vi "USBCam+Stage.vi"() -> ()   [LabVIEW 2014]
doc: "This is the main user interface of the Raman spectroscopy system."
uses:
  TypeDef/States.ctl
  C:/Users/light/Desktop/SI+Raman/Labview/Raman/dll/Thorlabs.MotionControl.Controls.dll
  dll/Thorlabs.MotionControl.Controls.dll
  C:/Users/light/Desktop/SI+Raman/Labview/Raman/dll/ThorLabs.MotionControl.KCube.DCServoCLI.dll
  dll/ThorLabs.MotionControl.KCube.DCServoCLI.dll
  TypeDef/StageDeviceOut.ctl
  TypeDef/StageHandleIn.ctl
  <vilib>/Utility/miscctls.llb/LVPoint32TypeDef.ctl
  TypeDef/StageSelect.ctl
  TypeDef/LaserSpot.ctl
panel:
  out "Spot Y":dbl
  out "Spot X":dbl
  in  "Box":cluster{"Width":dbl, " Height":dbl}={"Width"=200.0, " Height"=214.0}
  out "Total_Frame_Y":dbl
  out "Total_Frame_X":dbl
  out "Frame_Y":dbl
  out "Frame_X":dbl
  in  "Destination":dbl=12.0
  in  "Save Path":path=path "C:/Users/light/Desktop/Chuanzhen/test"
  in  "Scan":bool
  in  "Velocity: X and Y axis":T1(radio)=enum."0.05mm"
  in  "MoveTo":bool
  in  "Jogstep of Z axis":T2(radio)=enum."10step"
  in  "Z axis_d":bool
  in  "Z axis_u":bool
  in  "Y axis_F":bool
  in  "Y axis_B":bool
  out "Y_axis":dbl
  out "X_axis":dbl
  out "Z_axis":dbl
  in  "X axis_L":bool
  in  "X axis_R":bool
  in  "Down":bool
  in  "Top":bool
  in  "Right":bool
  in  "Left":bool
  in  "Snap":bool
  out "Boolean":bool
  in  "Pixel Size Y (um)":dbl=0.0877
  in  "LaserSpot":bool
  in  "Pixel Size X (um)":dbl=0.0877
  in  "Aim":bool
  out "Initialization finished":bool
  out "ZoomRatio":dbl format="%#_2g"
  out "Live video":picture caption="600 x 480"
  in  "Camera ID":u32
  out "Bits/Pixel":i32=8
  in  "Autogain":bool
  in  "Master Gain":i32(slide) min=0 max=100 scale=0.0..100.0
  in  "Hotpixel correction 2":bool
  in  "Blacklevel compensation":bool
  in  "Edge Filter":i32(ring)=2 items=["High"=1, "Low"=2]
  in  "Edge Filter Enable / Disable":bool
  in  "Exposure time (ms)":dbl(slide)=11.094175438596492 min=0.008982456140350877 max=101.68743859649123 step=0.05487719298245614 scale=0.008982456140350877..101.68743859649123 scale format="%#.3g"
  in  "Pixel clock":i32(slide)=20 min=7 max=86 scale=7.0..86.0
  in  "Frame rate":dbl(slide)=9.827169720568149 min=0.5 max=17.288905497022668 step=5.487719298245614e-05 scale=0.5..17.288905497022668 scale format="%^#_3g"
  in  "Blacklevel Offset":i32(slide) min=0 max=255 scale=0.0..255.0
  out "FPS":dbl=6.258409738085552
  out "Width":i32=640
  out "Height":i32=480
  in  "Stage Control":enum32{"X axis", "Y axis", "Z axis"}(tab)
  in  "X axis":refnum<k24>(container)
  in  "Y axis":refnum<k24>(container)
  in  "Quit":bool
  # "Camera Control"
  # "Objective: CFI Plan Fluor ELWD 60x (1.27 NA) \nThe depth of field: 1.78 um\nPixel Size: 0.0877um/px"
  # "Attention: \ndon't click button very fast"
  # "Motor Control"
  # "Aim"
  # "Adjust laser spot lightly"
  # "Stage Scan"
  # "Total_Frame"
  # "Current_Frame"
  # "X"
  # "Y"
  # "Focus distance ia about 2mm"
  # "Stepsize:"
  # "Jogstep:"
  # "0.00003mm/step"
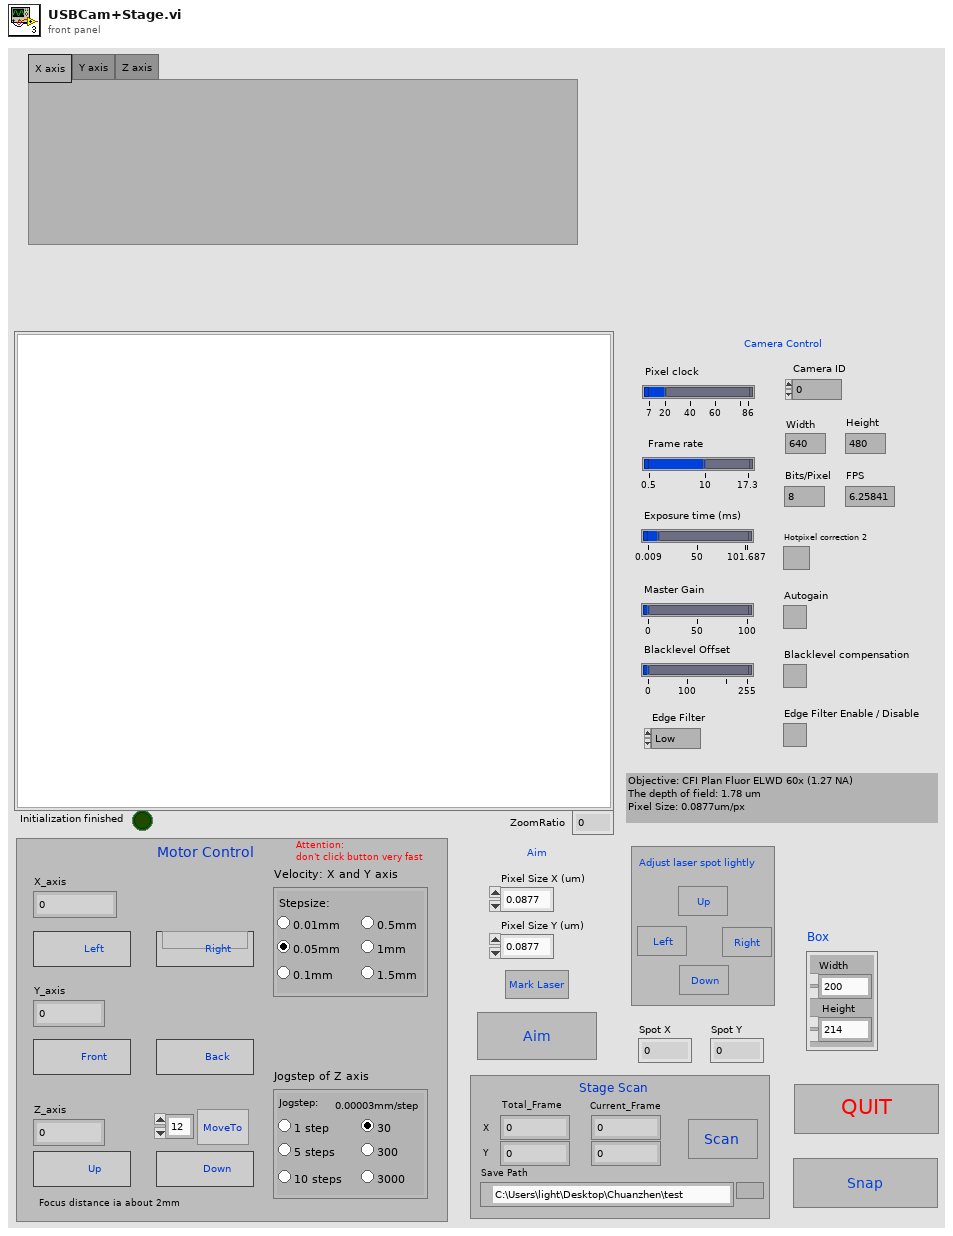
[diagram p1: front panel]
types:
  T1 = enum32{"0.01mm", "0.05mm", "0.1mm", "0.5mm", "1mm", "1.5mm"}
  T2 = enum32{"1step", "2step", "5step", "10step", "15step", "20step"}
  T3 = typedef "LaserSpot.ctl" = cluster{"Laser X":dbl, "Laser Y":dbl}
  T4 = cluster{"left":i16, "top":i16, "right":i16, "bottom":i16}
  T5 = typedef "LVPoint32TypeDef.ctl" = cluster{"Horizontal":i32, "Vertical":i32}
  T6 = typedef "StageHandleIn.ctl" = cluster{"X StageHandle in":refnum<k24>, "Y StageHandle in":refnum<k24>}
  T7 = typedef "StageDeviceOut.ctl" = cluster{"Device X":refnum<k24>, "Device Y":refnum<k24>}
  T8 = typedef "States.ctl" = enum16{"Initialize", "CMOS live", "Shut down"}
  T9 = cluster{"Width":u16, "Style":enum32{"Solid", "Dash", "Dot", "DashDot", "DashDotDot"}}
  T10 = typedef "StageSelect.ctl" = enum16{"X axis", "Y axis", "Z axis"}
  T11 = typedef "StageHandleOut.ctl" = cluster{"X StageHandle out":refnum<k24>, "Y StageHandle out":refnum<k24>}
  T12 = typedef "LVBoundsTypeDef.ctl" = cluster{"Width":u32, "Height":u32}
  T13 = typedef "imagedata.ctl" = cluster{"image type":i32, "image depth":i32, "image":u8[], "mask":u8[], "colors":u32[], "Rectangle":cluster{"left":i16, "top":i16, "right":i16, "bottom":i16}}
  T14 = typedef "LVPositionTypeDef.ctl" = cluster{"Left":i32, "Top":i32}
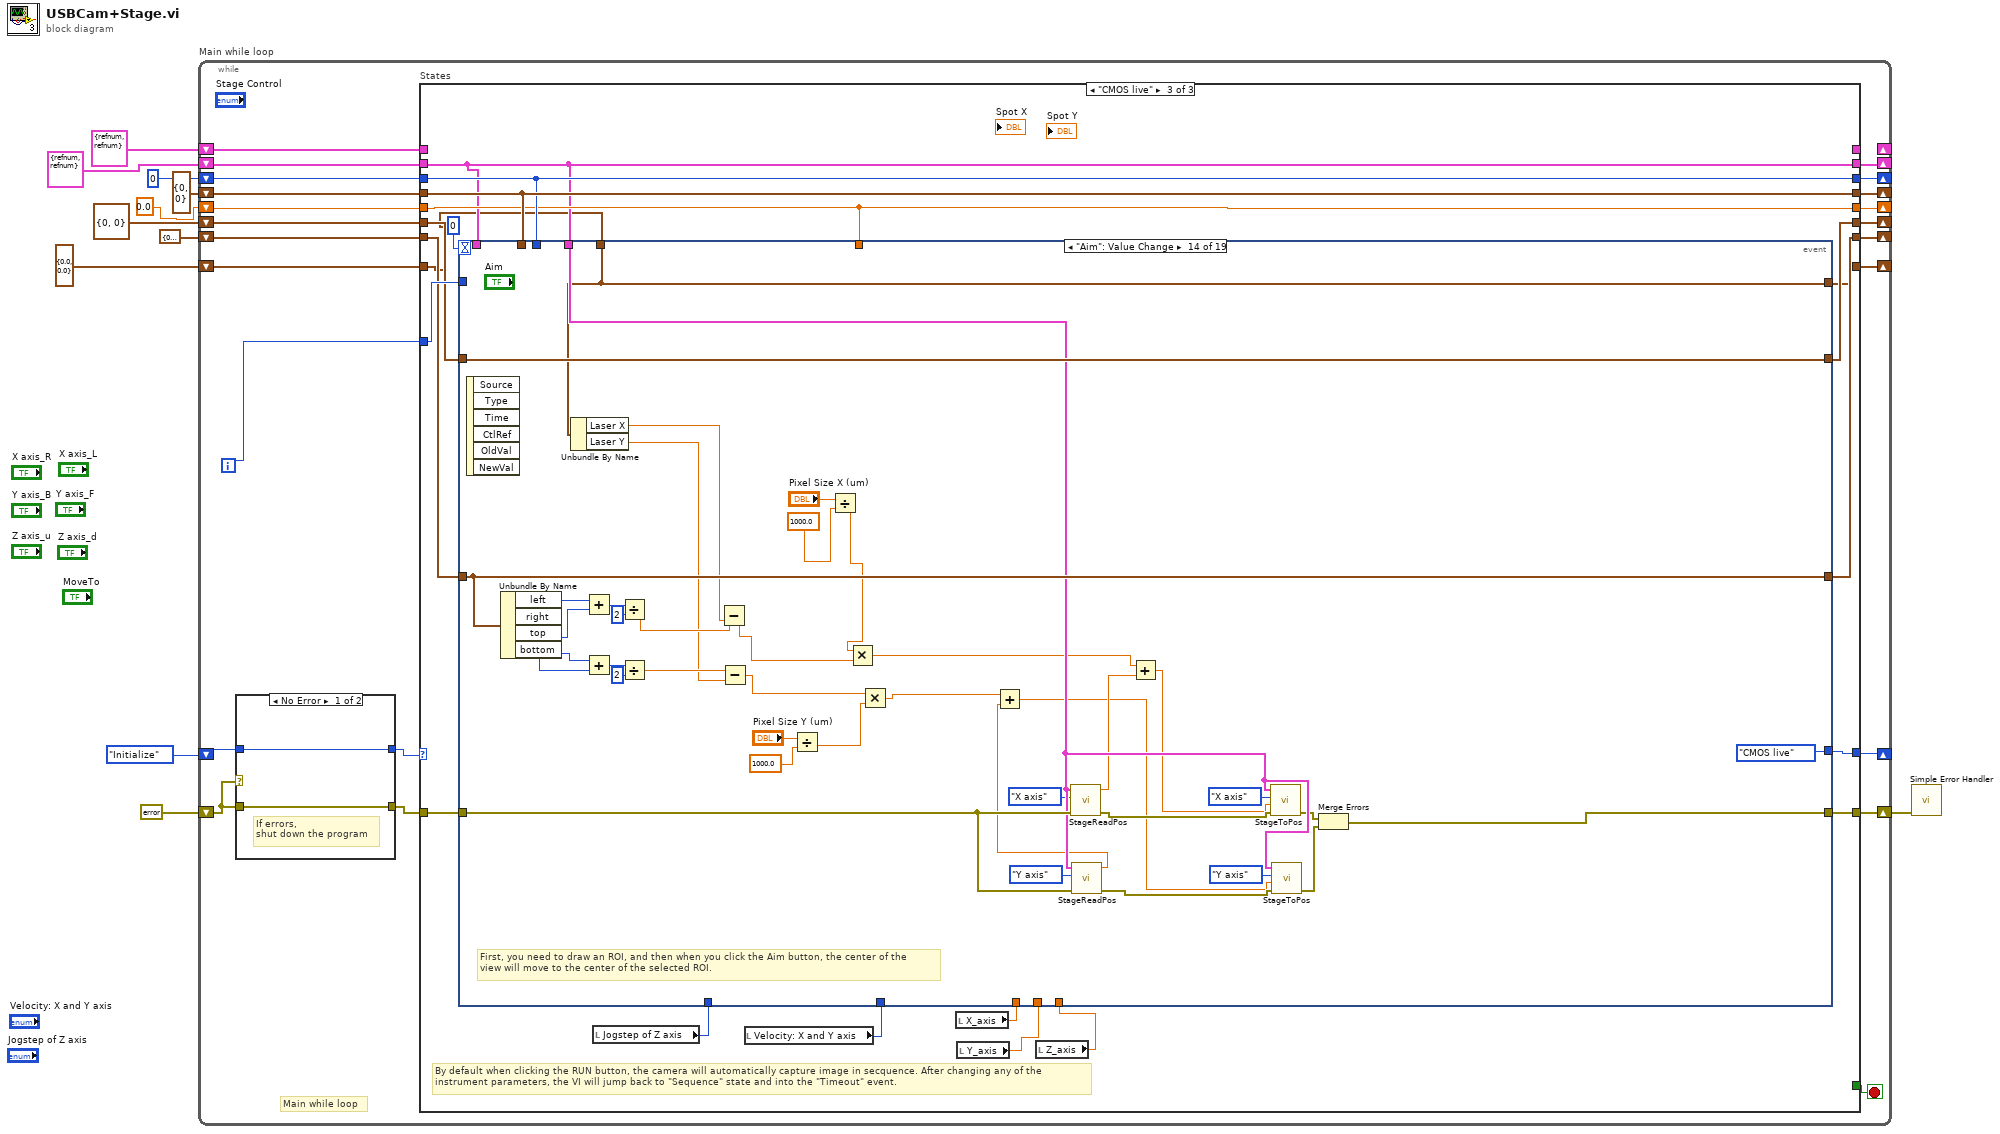
[diagram p0: block diagram]
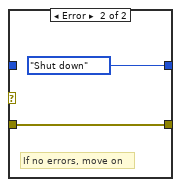
[diagram p2: hidden frame]
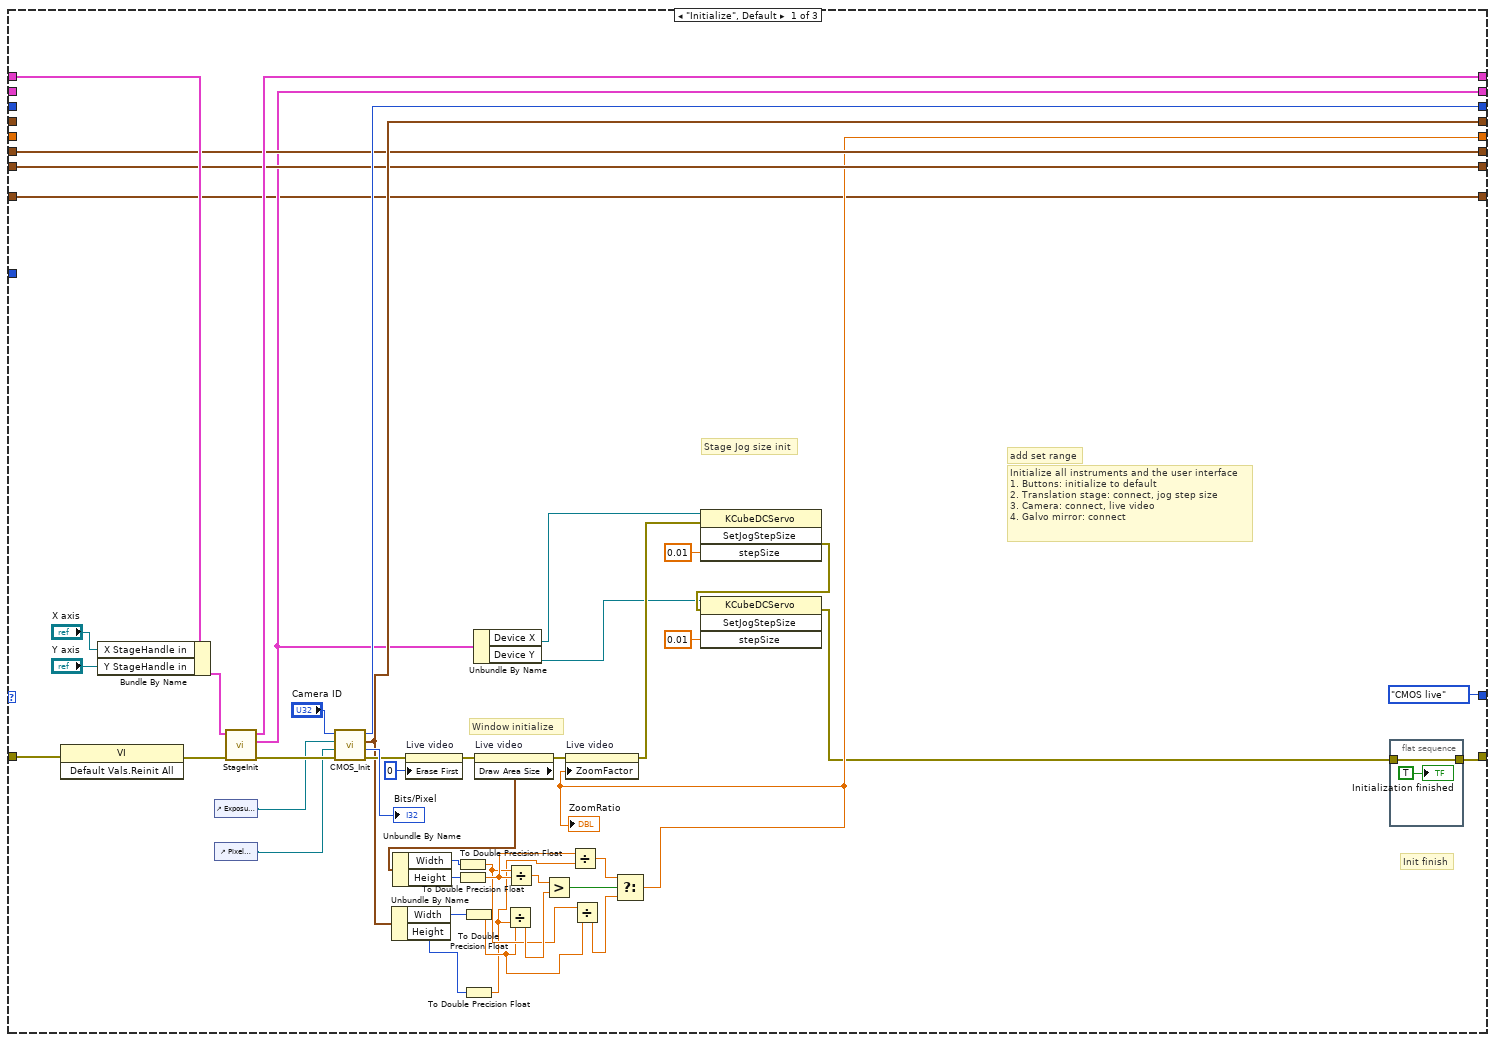
[diagram p3: hidden frame]
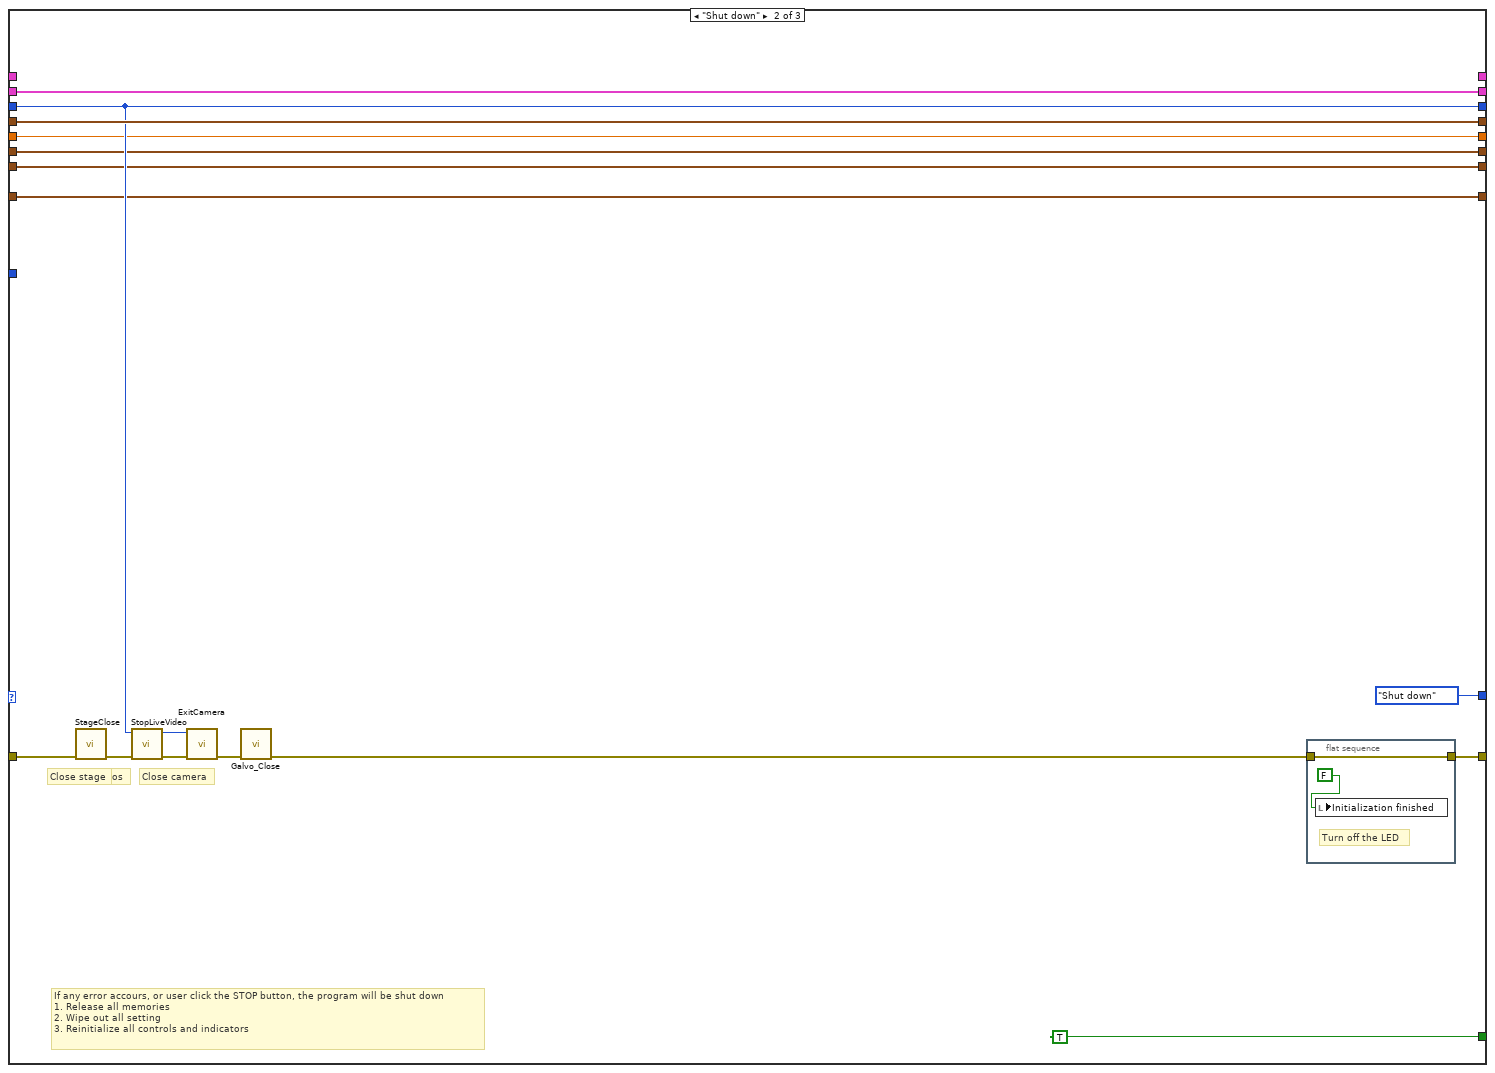
[diagram p4: hidden frame]
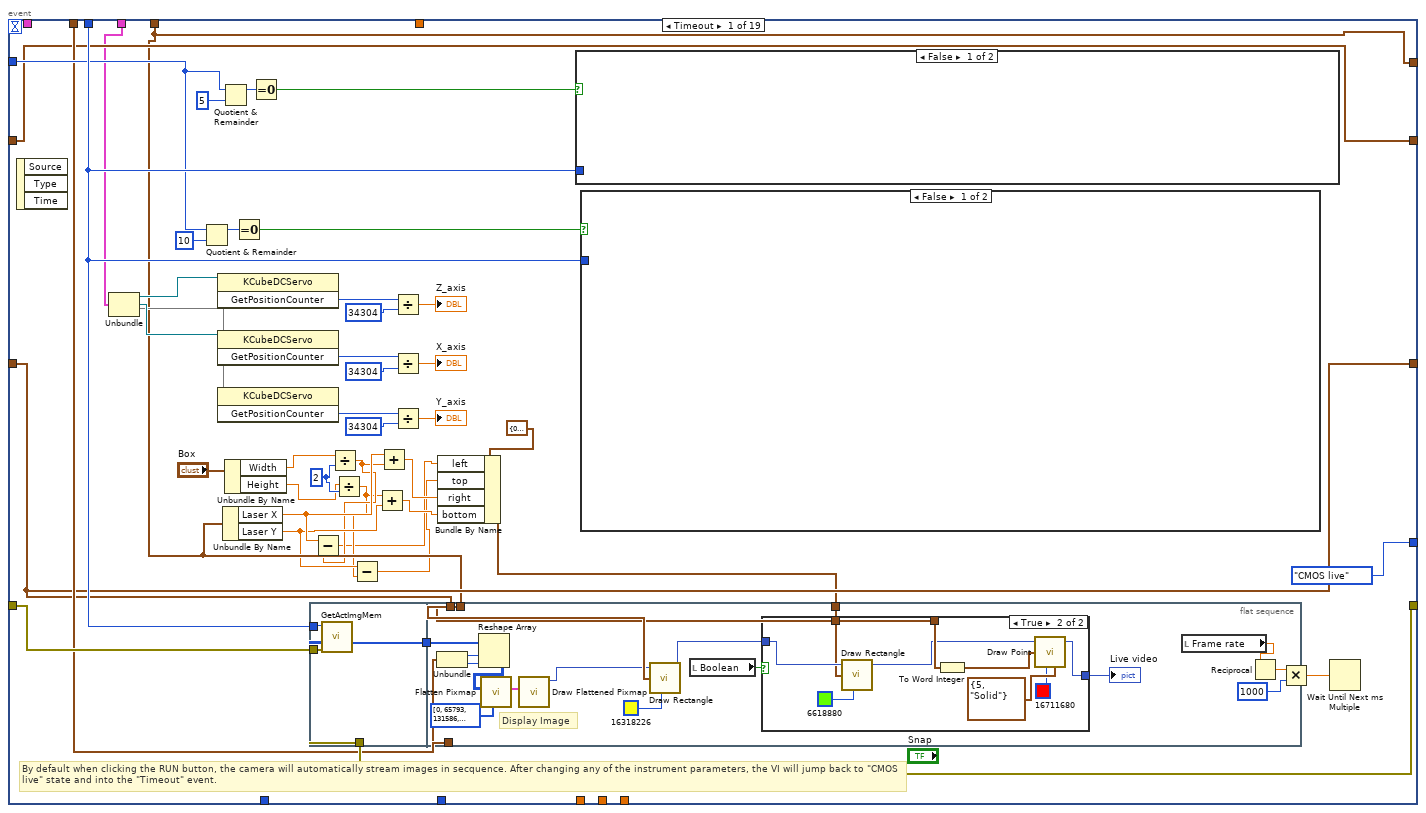
[diagram p5: hidden frame]
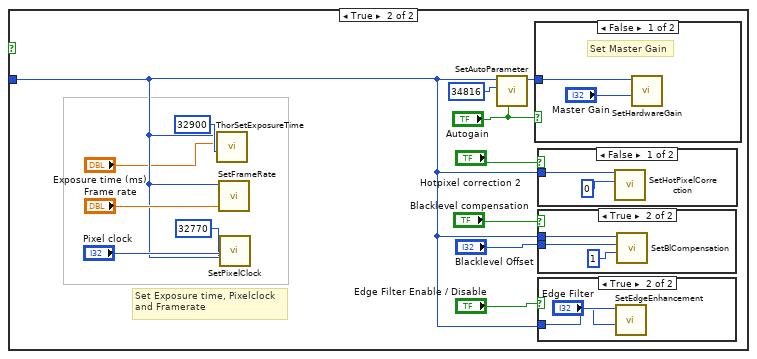
[diagram p6: hidden frame]
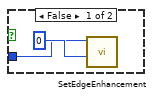
[diagram p7: hidden frame]
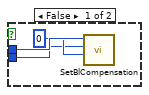
[diagram p8: hidden frame]
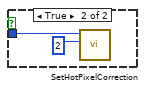
[diagram p9: hidden frame]
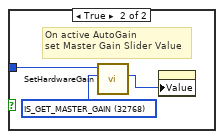
[diagram p10: hidden frame]
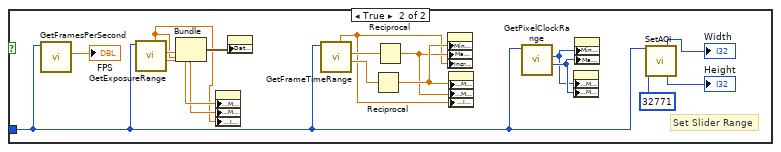
[diagram p11: hidden frame]
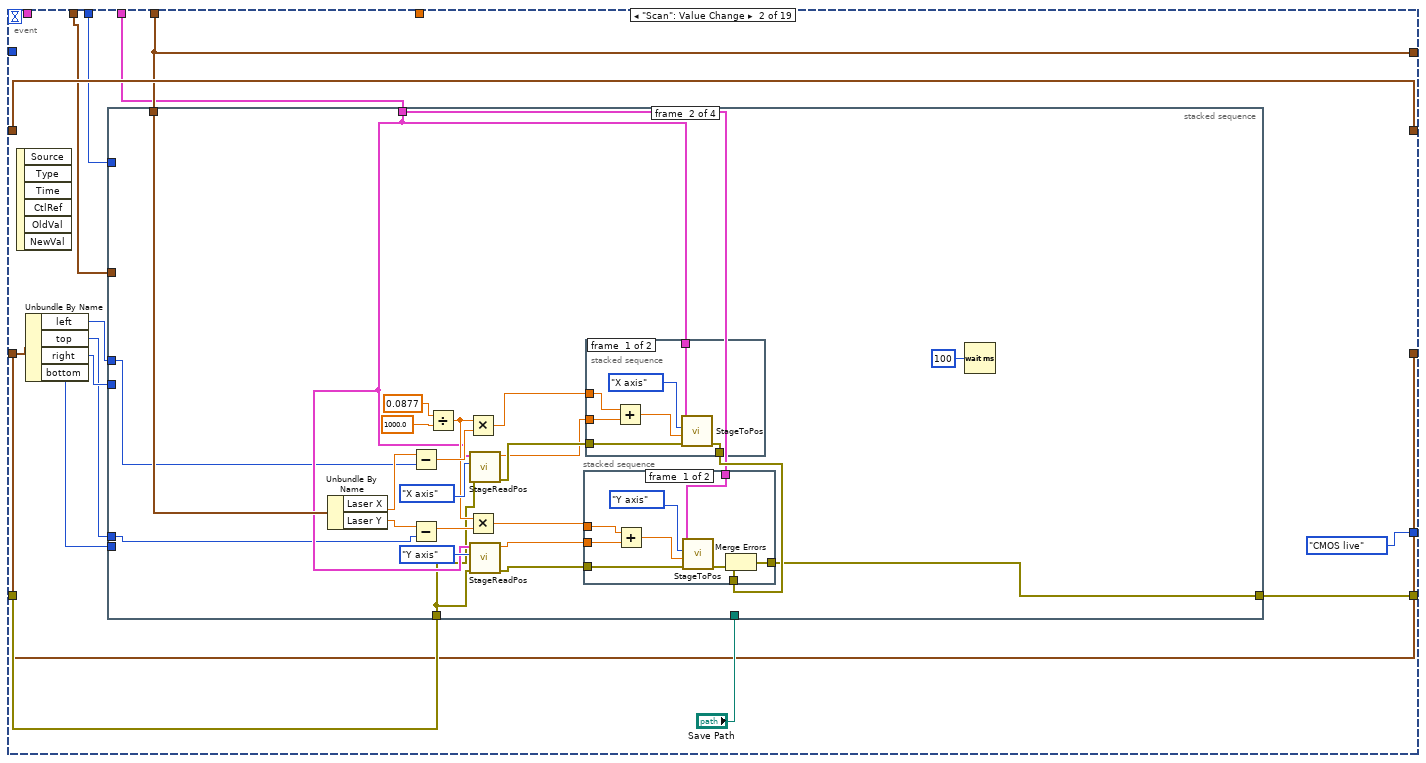
[diagram p13: hidden frame]
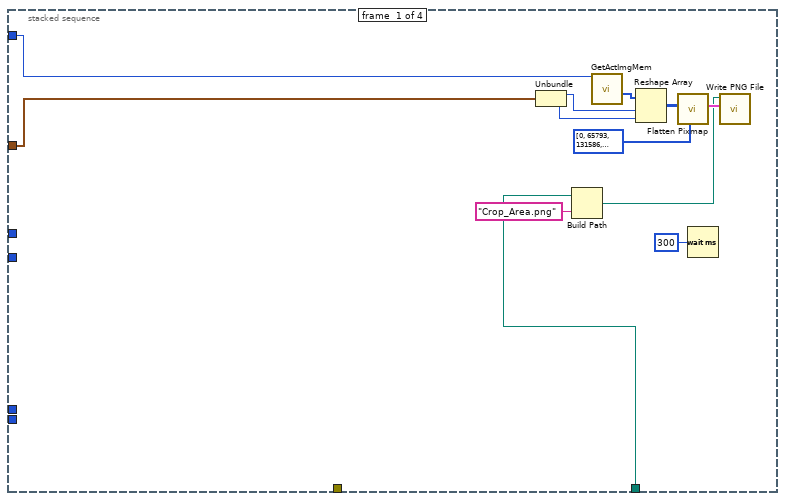
[diagram p14: hidden frame]
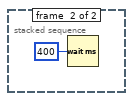
[diagram p15: hidden frame]
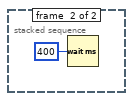
[diagram p16: hidden frame]
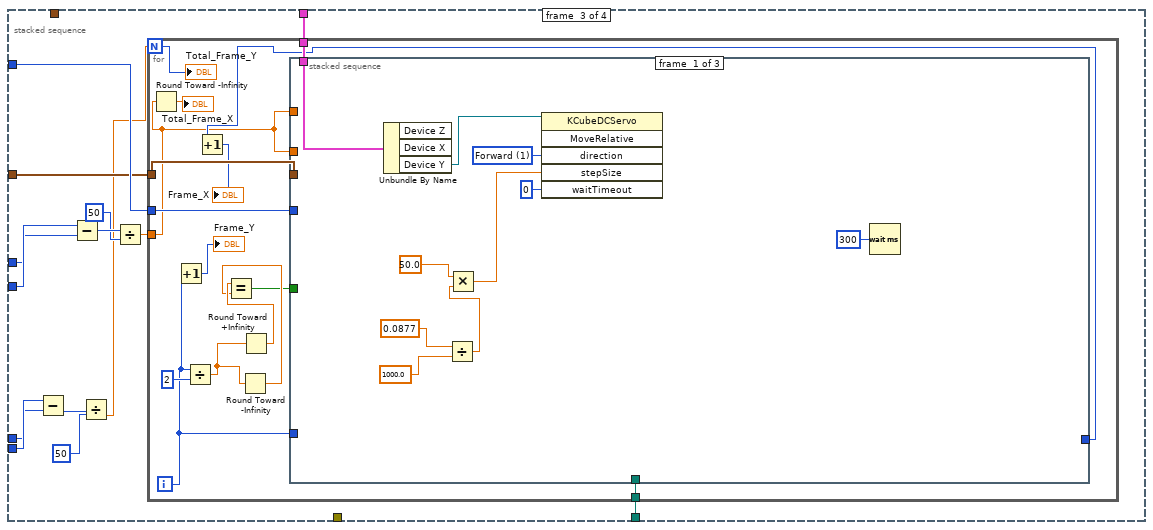
[diagram p17: hidden frame]
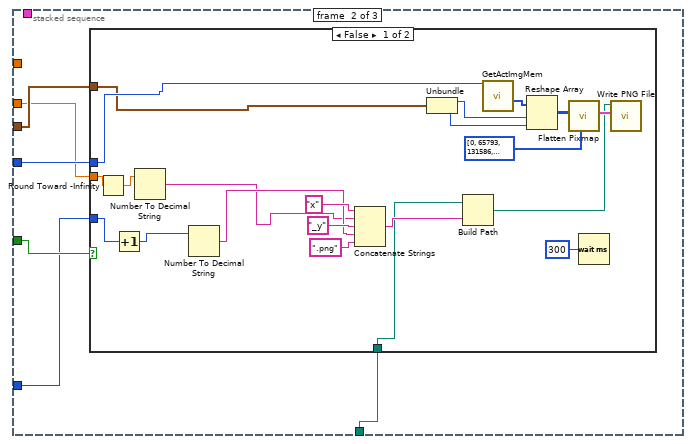
[diagram p18: hidden frame]
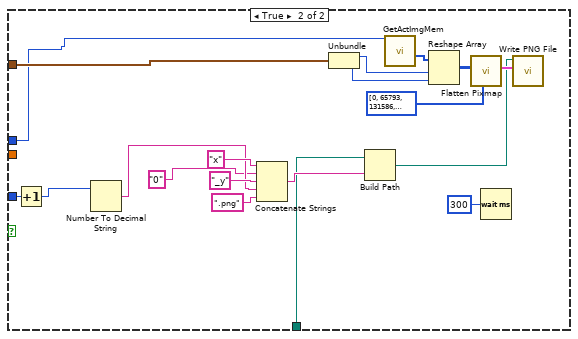
[diagram p19: hidden frame]
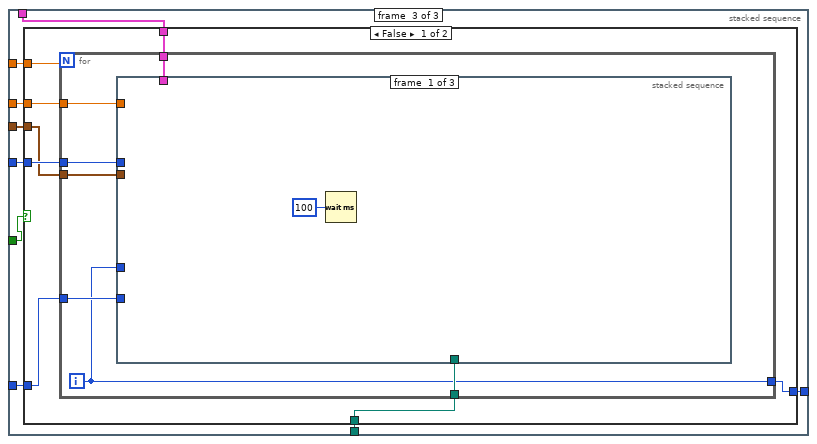
[diagram p20: hidden frame]
diagram:
  n1 = while "Main while loop" {
    shift-right: [w29] -> _
    shift-left: States."Initialize" -> [w34]
    shift-right: [w32] -> w9
    shift-left: errorcluster {"status"=FALSE, "code"=0, "source"=""} ("error out") -> [w28]
    shift-right: _ -> [_]
    shift-left: T6 {"X StageHandle in"=refnum, "Y StageHandle in"=refnum} ("StageHandle In") -> [w27]
    shift-right: [w26] -> _
    shift-left: T7 {"Device X"=refnum, "Device Y"=refnum} ("Device Out") -> [w25]
    shift-right: [w24] -> _
    shift-left: u32 0 ("CMOS Handle Out") -> [w23]
    shift-right: [w21] -> _
    shift-left: cluster{"Height":i32, "Width":i32} {"Height"=0, "Width"=0} ("WidthAndHeight") -> [w20]
    shift-right: [w19] -> _
    shift-left: 0.0 -> [w14]
    shift-right: [w18] -> _
    shift-left: T5 {"Horizontal"=0, "Vertical"=0} ("Coords") -> [w17]
    shift-right: [w16] -> _
    shift-left: T4 {"left"=0, "top"=0, "right"=0, "bottom"=0} ("rect") -> [w15]
    shift-right: [w13] -> _
    shift-left: T3 {"Laser X"=0.0, "Laser Y"=0.0} ("LaserSpot 2") -> [w12]
    i -> [w22]
    stop <- w30 stop-if-true
    # "Main while loop"
    n2 = case shown="No Error" w28 {
      tunnel: w28 -> [w36 w38]
      tunnel: [w36 w38] -> w31
      tunnel: w34 -> [w35 _]
      tunnel: [w35 States."Shut down"] -> w33
      frame No Error {
        # "If errors,\nshut down the program"
      }
      frame Error {
        # "If no errors, move on"
      }
    }
    n3 = case "States" shown="\"CMOS live\"" w33 {
      tunnel: [w39 w90 w122] -> w32
      tunnel: w31 -> [w83 w99 w123]
      tunnel: [_ TRUE _] -> w30
      tunnel: [States."CMOS live" States."Shut down" w124] -> w29
      tunnel: w27 -> [w81 _ _]
      tunnel: [w80 _ _] -> _
      tunnel: [w48 w100 w112] -> w26
      tunnel: w25 -> [_ w100 w112]
      tunnel: [w75 w94 w118] -> w24
      tunnel: w23 -> [_ w94 w118]
      tunnel: w22 -> [_ _ w120]
      tunnel: [w56 w98 w119] -> w21
      tunnel: w20 -> [_ w98 w119]
      tunnel: [w49 w93 w113] -> w19
      tunnel: w14 -> [_ w93 w113]
      tunnel: [w51 w92 w117] -> w18
      tunnel: w17 -> [w51 w92 w116]
      tunnel: [w50 w91 w115] -> w16
      tunnel: w15 -> [w50 w91 w114]
      tunnel: [w41 w87 w111] -> w13
      tunnel: w12 -> [w41 w87 w110]
      frame "Initialize", Default {
        # "Init finish"
        # "add set range"
        # "Stage Jog size init"
        # "Window initialize"
        # "Initialize all instruments and the user interface\n1. Buttons: initialize to default\n2. Translation stage: connect, jog step size\n3. Camera: connect, live video\n4. Galvo mirror: connect"
        n4 = invoke class="VI" method="Default Vals.Reinit All"(error in=w83) -> (error out=w82:errorcluster)  [unwired: 2 in, 2 out]
        n5 = Bundle By Name(cluster=w81, "X StageHandle in"="X axis", "Y StageHandle in"="Y axis") -> (w79:T6)
        n6 = control-ref of="Exposure time (ms)"() -> (w74:refnum<vi>)
        n7 = control-ref of="Pixel clock"() -> (w73:refnum<vi>)
        n8 = call "StageInit.vi"("error in (no error)"=w82, "StageHandle In"=w79) -> ("error out"=w76:errorcluster, "Device Out"=w48:T7, "StageHandle Out"=w80:T11)  [unwired: 7 in]
        n9 = call "CMOS_Init.vi"("error in"=w76, "Pixel clock"=w73, "Exposure time"=w74, "Camera ID"="Camera ID") -> ("error out"=w70:errorcluster, "Bits/Pixel"=→"Bits/Pixel":i32, "WidthAndHeight"=w56:cluster{"Height":i32, "Width":i32}, "CMOS Handle Out"=w75:u32)  [unwired: 3 in]
        n10 = Unbundle By Name(w56) -> ("Width"=w55:i32, "Height"=w54:i32)
        n11 = property on="Live video" class="Pict"(error in=w70, "Erase First"=u8 0) -> (error out=w58:errorcluster)  [unwired: 1 in, 1 out]
        n12 = To Double Precision Float(number=w55) -> (double precision float=w53:dbl)
        n13 = To Double Precision Float(number=w54) -> (double precision float=w52:dbl)
        n14 = Unbundle By Name(w48) -> ("Device X"=w43:refnum<k24>, "Device Y"=w42:refnum<k24>)
        n15 = property on="Live video" class="Pict"(error in=w58) -> (error out=w57:errorcluster, "Draw Area Size"=w68:T12)  [unwired: 1 in, 1 out]
        n16 = Unbundle By Name(w68) -> ("Width"=w66:u32, "Height"=w67:u32)
        n17 = To Double Precision Float(number=w66) -> (double precision float=w60:dbl)
        n18 = To Double Precision Float(number=w67) -> (double precision float=w62:dbl)
        n19 = Divide(x=w53, y=w52) -> (x/y=w63:dbl)
        n20 = Divide(x=w60, y=w62) -> (x/y=w65:dbl)
        n21 = Greater?(x=w65, y=w63) -> (0:w64:bool)
        n22 = Divide(x=w62, y=w52) -> (x/y=w61:dbl)
        n23 = Divide(x=w60, y=w53) -> (x/y=w59:dbl)
        n24 = Select(t=w61, s=w64, f=w59) -> (s? t:f=w49:dbl)
        "ZoomRatio" <- w49
        n25 = property on="Live video" class="Pict"(error in=w57, "ZoomFactor"=w49) -> (error out=w45:errorcluster)  [unwired: 1 in, 1 out]
        n26 = invoke class="KCubeDCServo" method="SetJogStepSize"(reference=w43, error in=w45, "stepSize"=0.01) -> (error out=w44:errorcluster)  [unwired: 1 in, 3 out]
        n27 = invoke class="KCubeDCServo" method="SetJogStepSize"(reference=w42, error in=w44, "stepSize"=0.01) -> (error out=w40:errorcluster)  [unwired: 1 in, 3 out]
        n28 = flat-sequence {
          tunnel: w40 -> [w85]
          tunnel: [w85] -> w39
          frame #0 {
            "Initialization finished" <- TRUE ("Initialization finished")
          }
        }
      }
      frame "Shut down" {
        # "Close 3 galvos"
        # "Close camera"
        # "Close stage"
        # "If any error accours, or user click the STOP button, the program will be shut down\n1. Release all memories\n2. Wipe out all setting\n3. Reinitialize all controls and indicators"
        n29 = call "StageClose.vi"("error in (no error)"=w99) -> ("error out"=w97:errorcluster)  [unwired: 10 in]
        n30 = call "StopLiveVideo.vi"("error in"=w97, "Camera Handle In"=w94) -> ("error out"=w96:errorcluster, "Camera Handle Out"=w95:u32)  [unwired: 8 in]
        n31 = call "ExitCamera.vi"("error in"=w96, "Camera Handle In"=w95) -> ("error out"=w89:errorcluster)  [unwired: 9 in]
        n32 = call "Galvo_Close.vi"("error in"=w89) -> ("error out"=w88:errorcluster)  [unwired: 10 in]
        n33 = flat-sequence {
          tunnel: w88 -> [w104]
          tunnel: [w104] -> w90
          frame #0 {
            # "Turn off the LED"
            n34 = local write "Initialization finished"(FALSE ("Initialization finished")) -> ()
          }
        }
      }
      frame "CMOS live" {
        # "By default when clicking the RUN button, the camera will automatically capture image in secquence. After changing any of the \ninstrument parameters, the VI will jump back to \"Sequence\" state and into the \"Timeout\" event."
        n35 = local read "Jogstep of Z axis"() -> (w105:T2)
        n36 = local read "Velocity: X and Y axis"() -> (w109:T1)
        n37 = local read "X_axis"() -> (w108:dbl)
        n38 = local read "Y_axis"() -> (w107:dbl)
        n39 = local read "Z_axis"() -> (w106:dbl)
        n40 = event shown="[13] \"Aim\": Value Change" {
          selector: _ -> [_ _ _ _ _ _ _ _ _ _ _ _ _ _ _ _ _ _ _]
          dyn-events: _ -> [_ _ _ _ _ _ _ _ _ _ _ _ _ _ _ _ _ _ _]
          timeout: 0 -> [_ _ _ _ _ _ _ _ _ _ _ _ _ _ _ _ _ _ _]
          tunnel: [States."CMOS live" States."CMOS live" States."CMOS live" States."CMOS live" States."CMOS live" States."CMOS live" States."CMOS live" States."CMOS live" States."CMOS live" States."CMOS live" States."CMOS live" States."CMOS live" States."Shut down" States."CMOS live" States."CMOS live" States."CMOS live" States."CMOS live" States."CMOS live" States."CMOS live"] -> w124
          tunnel: w123 -> [w160 w254 w521 w543 w567 w589 w613 w636 w655 w656 w670 w677 w708 w747 w767 w777 w787 w797 w807]
          tunnel: [w159 w253 w521 w543 w567 w589 w613 w636 w655 w656 w670 w677 w708 w748 w767 w777 w787 w797 w807] -> w122
          tunnel: w118 -> [w158 w252 _ _ _ _ _ _ _ w665 _ _ _ _ _ _ _ _ _]
          tunnel: w120 -> [w157 _ _ _ _ _ _ _ _ _ _ _ _ _ _ _ _ _ _]
          tunnel: w119 -> [w156 w251 _ _ _ _ _ _ _ w658 _ _ _ _ _ _ _ _ _]
          tunnel: [w154 w262 w520 w542 w566 w588 w612 w635 w654 w668 w672 w679 w707 w750 w766 w776 w786 w796 w806] -> w117
          tunnel: w116 -> [w154 w262 w520 w542 w566 w588 w612 w635 w654 w668 _ w679 w707 w750 w766 w776 w786 w796 w806]
          tunnel: [w155 w249 w519 w541 w565 w587 w611 w634 w653 w667 w671 w682 w706 w746 w756 w775 w785 w795 w805] -> w115
          tunnel: w114 -> [w155 w249 w519 w541 w565 w587 w611 w634 w653 w667 w671 _ w706 w746 w756 w775 w785 w795 w805]
          tunnel: w113 -> [_ _ _ _ _ _ _ _ _ _ _ w681 _ _ _ _ _ _ _]
          tunnel: w112 -> [_ _ _ _ _ _ _ _ _ _ _ _ _ _ _ _ _ _ _]
          tunnel: w112 -> [w152 w255 w517 w538 w560 w583 w605 w629 w647 _ _ _ _ w735 _ _ _ _ _]
          tunnel: [w137 w260 w518 w540 w564 w586 w610 w633 w652 w666 w669 w676 w705 w712 w754 w772 w780 w791 w801] -> w111
          tunnel: w110 -> [w137 w260 w518 w540 w564 w586 w610 w633 w652 w666 w669 w676 w705 w712 _ w771 w781 w792 w802]
          tunnel: w109 -> [_ _ w509 w533 w556 w579 _ _ _ _ _ _ _ _ _ _ _ _ _]
          tunnel: w108 -> [_ _ w512 w536 _ _ _ _ _ _ _ _ _ _ _ _ _ _ _]
          tunnel: w107 -> [_ _ _ _ w558 w581 _ _ _ _ _ _ _ _ _ _ _ _ _]
          tunnel: w106 -> [_ _ _ _ _ _ w602 w625 _ _ _ _ _ _ _ _ _ _ _]
          tunnel: w105 -> [_ _ _ _ _ _ w606 w628 _ _ _ _ _ _ _ _ _ _ _]
          event Timeout {
            w136 = 2
            # "By default when clicking the RUN button, the camera will automatically stream images in secquence. After changing any of the instrument parameters, the VI will jump back to \"CMOS live\" state and into the \"Timeout\" event."
            n41 = event-data() -> ()  [unwired: 1 in, 3 out]
            n42 = Unbundle(w152) -> (w142:refnum<k24>, w141:refnum<k24>, w140)
            n43 = Quotient & Remainder(x=w157, y=10) -> (x-y*floor(x/y)=w167:i32)  [unwired: 1 out]
            n44 = invoke class="KCubeDCServo" method="GetPositionCounter"(reference=w142) -> ("GetPositionCounter"=w151:i32)  [unwired: 2 in, 2 out]
            n45 = invoke class="KCubeDCServo" method="GetPositionCounter"(reference=w141) -> ("GetPositionCounter"=w150:i32)  [unwired: 2 in, 2 out]
            n46 = invoke class="KCubeDCServo" method="GetPositionCounter"(reference=w140) -> ("GetPositionCounter"=w149:i32)  [unwired: 2 in, 2 out]
            n47 = Quotient & Remainder(x=w157, y=5) -> (x-y*floor(x/y)=w170:i32)  [unwired: 1 out]
            n48 = Unbundle By Name(w137) -> ("Laser X"=w131:dbl, "Laser Y"=w130:dbl)
            n49 = Unbundle By Name("Box") -> ("Width"=w135:dbl, "Height"=w134:dbl)
            n50 = Equal To 0?(x=w167) -> (x = 0?=w165:bool)
            n51 = Equal To 0?(x=w170) -> (x = 0?=w169:bool)
            n52 = flat-sequence {
              tunnel: [w222] -> w171
              tunnel: w158 -> [w223]
              tunnel: w160 -> [w221]
              tunnel: [w220] -> w159
              tunnel: w171 -> [w238]
              tunnel: w156 -> [w237]
              tunnel: w155 -> [w230]
              tunnel: w137 -> [w226]
              tunnel: w125 -> [w224]
              frame #0 {
                n53 = call "GetActImgMem.vi"("error in"=w221, "Camera Handle In"=w223) -> ("error out"=w220:errorcluster, "Image Memory Out"=w222:u8[])  [unwired: 6 in, 2 out]
              }
              frame #1 {
                # "Display Image"
                n54 = Unbundle(w237) -> ("Height"=w236:i32, "Width"=w235:i32)
                n55 = Reshape Array(w238, w236, w235) -> (w234:u8[][])
                n56 = call <vilib>:"Flatten Pixmap.vi"("colors"=u32[] [0, 65793, 131586, 197379, 263172, 328965, 394758, 460551, 526344, 592137, 657930, 723723, 789516, 855309, 921102, 986895, 1052688, 1118481, 1184274, 1250067, 1315860, 1381653, 1447446, 1513239, 1579032, 1644825, 1710618, 1776411, 1842204, 1907997, 1973790, 2039583, 2105376, 2171169, 2236962, 2302755, 2368548, 2434341, 2500134, 2565927, 2631720, 2697513, 2763306, 2829099, 2894892, 2960685, 3026478, 3092271, 3158064, 3223857, 3289650, 3355443, 3421236, 3487029, 3552822, 3618615, 3684408, 3750201, 3815994, 3881787, 3947580, 4013373, 4079166, 4144959, 4210752, 4276545, 4342338, 4408131, 4473924, 4539717, 4605510, 4671303, 4737096, 4802889, 4868682, 4934475, 5000268, 5066061, 5131854, 5197647, 5263440, 5329233, 5395026, 5460819, 5526612, 5592405, 5658198, 5723991, 5789784, 5855577, 5921370, 5987163, 6052956, 6118749, 6184542, 6250335, 6316128, 6381921, 6447714, 6513507, 6579300, 6645093, 6710886, 6776679, 6842472, 6908265, 6974058, 7039851, 7105644, 7171437, 7237230, 7303023, 7368816, 7434609, 7500402, 7566195, 7631988, 7697781, 7763574, 7829367, 7895160, 7960953, 8026746, 8092539, 8158332, 8224125, 8289918, 8355711, 8421504, 8487297, 8553090, 8618883, 8684676, 8750469, 8816262, 8882055, 8947848, 9013641, 9079434, 9145227, 9211020, 9276813, 9342606, 9408399, 9474192, 9539985, 9605778, 9671571, 9737364, 9803157, 9868950, 9934743, 10000536, 10066329, 10132122, 10197915, 10263708, 10329501, 10395294, 10461087, 10526880, 10592673, 10658466, 10724259, 10790052, 10855845, 10921638, 10987431, 11053224, 11119017, 11184810, 11250603, 11316396, 11382189, 11447982, 11513775, 11579568, 11645361, 11711154, 11776947, 11842740, 11908533, 11974326, 12040119, 12105912, 12171705, 12237498, 12303291, 12369084, 12434877, 12500670, 12566463, 12632256, 12698049, 12763842, 12829635, 12895428, 12961221, 13027014, 13092807, 13158600, 13224393, 13290186, 13355979, 13421772, 13487565, 13553358, 13619151, 13684944, 13750737, 13816530, 13882323, 13948116, 14013909, 14079702, 14145495, 14211288, 14277081, 14342874, 14408667, 14474460, 14540253, 14606046, 14671839, 14737632, 14803425, 14869218, 14935011, 15000804, 15066597, 15132390, 15198183, 15263976, 15329769, 15395562, 15461355, 15527148, 15592941, 15658734, 15724527, 15790320, 15856113, 15921906, 15987699, 16053492, 16119285, 16185078, 16250871, 16316664, 16382457, 16448250, 16514043, 16579836, 16645629, 16711422, 0] ("output array 2"), "8-bit pixmap"=w234) -> ("image data"=w233:T13)  [unwired: 9 in]
                n57 = call <vilib>:"Draw Flattened Pixmap.vi"("image data"=w233) -> ("new picture"=w225:picture)  [unwired: 8 in]
                n58 = call <vilib>:"Draw Rectangle.vi"("picture"=w225, "rect"=w230, "color(black)"=u32 16318226) -> ("new picture"=w229:picture)  [unwired: 6 in]
                n59 = local read "Boolean"() -> (w227:bool)
                n60 = case shown="True" w227 {
                  tunnel: w229 -> [w239 w243]
                  tunnel: [w239 w245] -> w228
                  tunnel: w226 -> [_ w244]
                  tunnel: w224 -> [_ w241]
                  frame False {
                  }
                  frame True {
                    n61 = call <vilib>:"Draw Rectangle.vi"("picture"=w243, "rect"=w241, "color(black)"=u32 6618880) -> ("new picture"=w242:picture)  [unwired: 6 in]
                    n62 = To Word Integer(number=w244) -> (16bit integer=w246:cluster{"Laser X":i16, "Laser Y":i16})
                    n63 = call <vilib>:"Draw Point.vi"("picture"=w242, "point(x,y)"=w246, "color(black)"=u32 16711680, "pen"=T9 {"Width"=5, "Style"=enum."Solid"}) -> ("new picture"=w245:picture)  [unwired: 5 in]
                  }
                }
                "Live video" <- w228
              }
            }
            n64 = Divide(x=w135, y=w136) -> (x/y=w129:dbl)
            n65 = Subtract(x=w131, y=w129) -> (x-y=w127:dbl)
            n66 = Divide(x=w134, y=w136) -> (x/y=w128:dbl)
            n67 = Subtract(x=w130, y=w128) -> (x-y=w126:dbl)
            n68 = Add(x=w128, y=w130) -> (x+y=w132:dbl)
            n69 = Add(x=w131, y=w129) -> (x+y=w133:dbl)
            n70 = Divide(x=w151, y=34304) -> (x/y=→"Z_axis":dbl)
            n71 = Divide(x=w150, y=34304) -> (x/y=→"X_axis":dbl)
            n72 = Divide(x=w149, y=34304) -> (x/y=→"Y_axis":dbl)
            n73 = Bundle By Name(cluster=T4 {"left"=0, "top"=0, "right"=0, "bottom"=0} ("rect"), "left"=w127, "top"=w126, "right"=w133, "bottom"=w132) -> (w125:T4)
            n74 = case shown="False" w169 {
              tunnel: w158 -> [_ w206]
              frame False {
              }
              frame True {
                # "Set Slider Range"
                n75 = call "GetFramesPerSecond.vi"("Camera Handle In"=w206) -> ("FPS"=→"FPS":dbl)  [unwired: 8 in, 2 out]
                n76 = call "GetExposureRange.vi"("Camera Handle In"=w206) -> ("max"=w216:dbl, "min"=w217:dbl, "intervall"=w215:dbl)  [unwired: 6 in, 2 out]
                n77 = Bundle("min"=w217, "max"=w216, "intervall"=w215) -> (w218:cluster{"min":dbl, "max":dbl, "intervall":dbl})  [unwired: 1 in]
                n78 = property on="Exposure time (ms)" class="Schieberegler (strikt)"("Scale.Minimum"=w217, "Scale.Maximum"=w216, "Scale.Increment"=w215) -> ()  [unwired: 2 in, 2 out]
                n79 = property on="Exposure time (ms)" class="Schieberegler (strikt)"("Data Range"=w218) -> ()  [unwired: 2 in, 2 out]
                n80 = call "GetFrameTimeRange.vi"("Camera Handle In"=w206) -> ("max"=w212:dbl, "min"=w211:dbl, "interval"=w208:dbl)  [unwired: 6 in, 2 out]
                n81 = Reciprocal(x=w212) -> (1/x=w210:dbl)
                n82 = Reciprocal(x=w211) -> (1/x=w209:dbl)
                n83 = property on="Frame rate" class="Schieberegler (strikt)"("Minimum"=w210, "Maximum"=w209, "Increment"=w208) -> ()  [unwired: 2 in, 2 out]
                n84 = property on="Frame rate" class="Schieberegler (strikt)"("Scale.Minimum"=w210, "Scale.Maximum"=w209, "Scale.Increment"=w208) -> ()  [unwired: 2 in, 2 out]
                n85 = call "GetPixelClockRange.vi"("Camera Handle In"=w206) -> ("Max"=w214:i32, "Min"=w213:i32)  [unwired: 7 in, 2 out]
                n86 = property on="Pixel clock" class="Schieberegler (strikt)"("Scale.Minimum"=w213, "Scale.Maximum"=w214) -> ()  [unwired: 2 in, 2 out]
                n87 = property on="Pixel clock" class="Schieberegler (strikt)"("Minimum"=w213, "Maximum"=w214) -> ()  [unwired: 2 in, 2 out]
                n88 = call "SetAOI.vi"("Camera Handle In"=w206, "Mode"=32771) -> ("Width Out"=→"Width":i32, "Height Out"=→"Height":i32)  [unwired: 8 in, 4 out]
              }
            }
            n89 = case shown="False" w165 {
              tunnel: w158 -> [_ w175]
              frame False {
              }
              frame True {
                # "Set Exposure time, Pixelclock\nand Framerate"
                n90 = call "ThorSetExposureTime.vi"("Mode"=u16 32900, "Exposure Time"="Exposure time (ms)", "Camera Handle In"=w175) -> ()  [unwired: 6 in, 3 out]
                n91 = call "SetFrameRate.vi"("FPS"="Frame rate", "Camera Handle In"=w175) -> ()  [unwired: 7 in, 3 out]
                n92 = call "SetPixelClock.vi"("Mode"=32770, "Pixel Clock"="Pixel clock", "Camera Handle In"=w175) -> ()  [unwired: 6 in, 3 out]
                n93 = call "SetAutoParameter.vi"("enable"="Autogain", "Param"=34816, "Camera Handle In"=w175) -> ("Camera Handle Out"=w183:u32)  [unwired: 6 in, 2 out]
                n94 = case shown="False" "Autogain" {
                  tunnel: w183 -> [w199 w202]
                  frame False {
                    # "Set Master Gain"
                    n95 = call "SetHardwareGain.vi"("Master Gain"="Master Gain", "Camera Handle In"=w199) -> ()  [unwired: 7 in, 3 out]
                  }
                  frame True {
                    w201 = 32768 items=["IS_GET_MASTER_GAIN"=32768]
                    # "On active AutoGain\nset Master Gain Slider Value"
                    n96 = call "SetHardwareGain.vi"("Mode"=w201, "Camera Handle In"=w202) -> ("Value"=w203:i32)  [unwired: 7 in, 2 out]
                    n97 = property on="Master Gain" class="Slide (strict)"("Value"=w203) -> ()  [unwired: 2 in, 2 out]
                  }
                }
                n98 = case shown="False" "Hotpixel correction 2" {
                  tunnel: w175 -> [w196 w198]
                  frame False {
                    n99 = call "SetHotPixelCorrection.vi"("Mode"=0, "Camera Handle In"=w196) -> ()  [unwired: 7 in, 3 out]
                  }
                  frame True {
                    n100 = call "SetHotPixelCorrection.vi"("Mode"=2, "Camera Handle In"=w198) -> ()  [unwired: 7 in, 3 out]
                  }
                }
                n101 = case shown="True" "Blacklevel compensation" {
                  tunnel: w175 -> [w191 w194]
                  tunnel: "Blacklevel Offset" -> [w189 w192]
                  frame False {
                    n102 = call "SetBlCompensation.vi"("Mode"=0, "offset"=w189, "Camera Handle In"=w191) -> ()  [unwired: 6 in, 3 out]
                  }
                  frame True {
                    n103 = call "SetBlCompensation.vi"("Mode"=1, "offset"=w192, "Camera Handle In"=w194) -> ()  [unwired: 6 in, 3 out]
                  }
                }
                n104 = case shown="True" "Edge Filter Enable / Disable" {
                  tunnel: w175 -> [w185 w188]
                  frame False {
                    n105 = call "SetEdgeEnhancement.vi"("Mode"=0, "Camera Handle In"=w185) -> ()  [unwired: 8 in, 2 out]
                  }
                  frame True {
                    n106 = call "SetEdgeEnhancement.vi"("Mode"="Edge Filter", "Camera Handle In"=w188) -> ()  [unwired: 8 in, 2 out]
                  }
                }
              }
            }
            n107 = local read "Frame rate"() -> (w164:dbl)
            n108 = Reciprocal(x=w164) -> (1/x=w163:dbl)
            n109 = Multiply(x=w163, y=1000) -> (x*y=w161:dbl)
            n110 = Wait Until Next ms Multiple(millisecond multiple=w161) -> ()  [unwired: 1 out]
          }
          event "Scan": Value Change {
            n111 = event-data() -> ()  [unwired: 1 in, 6 out]
            n112 = Unbundle By Name(w249) -> ("left"=w259:i16, "top"=w257:i16, "right"=w258:i16, "bottom"=w256:i16)
            n113 = stacked-sequence {
              tunnel: w260 -> [_ w295 _ _]
              tunnel: w259 -> [_ w277 w328 _]
              tunnel: w258 -> [_ _ w329 _]
              tunnel: w257 -> [_ w276 w321 _]
              tunnel: w256 -> [_ _ w322 _]
              tunnel: w255 -> [_ w280 w320 _]
              tunnel: w254 -> [_ w279 _ _]
              tunnel: [_ w278 _ _] -> w253
              tunnel: w252 -> [w263 _ w319 _]
              tunnel: w251 -> [w264 _ w318 _]
              tunnel: "Save Path" -> [w266 _ w317 _]
              frame #0 {
                n114 = Unbundle(w264) -> ("Height"=w269:i32, "Width"=w268:i32)
                n115 = Build Path(base path=w266, name or relative path="Crop_Area.png") -> (appended path=w270:path)
                n116 = call "GetActImgMem.vi"("Camera Handle In"=w263) -> ("Image Memory Out"=w273:u8[])  [unwired: 7 in, 3 out]
                n117 = Reshape Array(w273, w269, w268) -> (w274:u8[][])
                n118 = call <vilib>:"Flatten Pixmap.vi"("colors"=u32[] [0, 65793, 131586, 197379, 263172, 328965, 394758, 460551, 526344, 592137, 657930, 723723, 789516, 855309, 921102, 986895, 1052688, 1118481, 1184274, 1250067, 1315860, 1381653, 1447446, 1513239, 1579032, 1644825, 1710618, 1776411, 1842204, 1907997, 1973790, 2039583, 2105376, 2171169, 2236962, 2302755, 2368548, 2434341, 2500134, 2565927, 2631720, 2697513, 2763306, 2829099, 2894892, 2960685, 3026478, 3092271, 3158064, 3223857, 3289650, 3355443, 3421236, 3487029, 3552822, 3618615, 3684408, 3750201, 3815994, 3881787, 3947580, 4013373, 4079166, 4144959, 4210752, 4276545, 4342338, 4408131, 4473924, 4539717, 4605510, 4671303, 4737096, 4802889, 4868682, 4934475, 5000268, 5066061, 5131854, 5197647, 5263440, 5329233, 5395026, 5460819, 5526612, 5592405, 5658198, 5723991, 5789784, 5855577, 5921370, 5987163, 6052956, 6118749, 6184542, 6250335, 6316128, 6381921, 6447714, 6513507, 6579300, 6645093, 6710886, 6776679, 6842472, 6908265, 6974058, 7039851, 7105644, 7171437, 7237230, 7303023, 7368816, 7434609, 7500402, 7566195, 7631988, 7697781, 7763574, 7829367, 7895160, 7960953, 8026746, 8092539, 8158332, 8224125, 8289918, 8355711, 8421504, 8487297, 8553090, 8618883, 8684676, 8750469, 8816262, 8882055, 8947848, 9013641, 9079434, 9145227, 9211020, 9276813, 9342606, 9408399, 9474192, 9539985, 9605778, 9671571, 9737364, 9803157, 9868950, 9934743, 10000536, 10066329, 10132122, 10197915, 10263708, 10329501, 10395294, 10461087, 10526880, 10592673, 10658466, 10724259, 10790052, 10855845, 10921638, 10987431, 11053224, 11119017, 11184810, 11250603, 11316396, 11382189, 11447982, 11513775, 11579568, 11645361, 11711154, 11776947, 11842740, 11908533, 11974326, 12040119, 12105912, 12171705, 12237498, 12303291, 12369084, 12434877, 12500670, 12566463, 12632256, 12698049, 12763842, 12829635, 12895428, 12961221, 13027014, 13092807, 13158600, 13224393, 13290186, 13355979, 13421772, 13487565, 13553358, 13619151, 13684944, 13750737, 13816530, 13882323, 13948116, 14013909, 14079702, 14145495, 14211288, 14277081, 14342874, 14408667, 14474460, 14540253, 14606046, 14671839, 14737632, 14803425, 14869218, 14935011, 15000804, 15066597, 15132390, 15198183, 15263976, 15329769, 15395562, 15461355, 15527148, 15592941, 15658734, 15724527, 15790320, 15856113, 15921906, 15987699, 16053492, 16119285, 16185078, 16250871, 16316664, 16382457, 16448250, 16514043, 16579836, 16645629, 16711422, 0] ("output array 2"), "8-bit pixmap"=w274) -> ("image data"=w271:T13)  [unwired: 9 in]
                n119 = Wait (ms)(milliseconds to wait=u32 300) -> ()  [unwired: 1 out]
                n120 = call <vilib>:"Write PNG File.vi"("image data"=w271, "path to PNG file"=w270) -> ()  [unwired: 8 in, 2 out]
              }
              frame #1 {
                n121 = Unbundle By Name(w295) -> ("Laser X"=w287:dbl, "Laser Y"=w286:dbl)
                n122 = Subtract(x=w287, y=w277) -> (x-y=w285:dbl)
                n123 = Subtract(x=w286, y=w276) -> (x-y=w283:dbl)
                n124 = Divide(x=0.0877, y=1000.0) -> (x/y=w284:dbl)
                n125 = Multiply(x=w284, y=w285) -> (x*y=w282:dbl)
                n126 = Multiply(x=w284, y=w283) -> (x*y=w281:dbl)
                n127 = call "StageReadPos.vi"("error in (no error)"=w279, "Stage Select"=StageSelect."X axis", "Device In"=w280) -> ("error out"=w294:errorcluster, "CurrentPosition"=w292:dbl)  [unwired: 7 in]
                n128 = call "StageReadPos.vi"("error in (no error)"=w279, "Stage Select"=StageSelect."Y axis", "Device In"=w280) -> ("error out"=w290:errorcluster, "CurrentPosition"=w289:dbl)  [unwired: 7 in]
                n129 = stacked-sequence {
                  tunnel: w294 -> [w314 _]
                  tunnel: w292 -> [w312 _]
                  tunnel: [w310 _] -> w288
                  tunnel: w282 -> [w309 _]
                  tunnel: w280 -> [w308 _]
                  frame #0 {
                    n130 = Add(x=w309, y=w312) -> (x+y=w311:dbl)
                    n131 = call "StageToPos.vi"("error in (no error)"=w314, "Move to pos"=w311, "Stage Select"=StageSelect."X axis", "Device In"=w308) -> ("error out"=w310:errorcluster)  [unwired: 7 in]
                  }
                  frame #1 {
                    n132 = Wait (ms)(milliseconds to wait=u32 400) -> ()  [unwired: 1 out]
                  }
                }
                n133 = stacked-sequence {
                  tunnel: w290 -> [w305 _]
                  tunnel: w289 -> [w304 _]
                  tunnel: w288 -> [w302 _]
                  tunnel: w281 -> [w300 _]
                  tunnel: w280 -> [w299 _]
                  tunnel: [w298 _] -> w278
                  frame #0 {
                    n134 = Add(x=w300, y=w304) -> (x+y=w303:dbl)
                    n135 = call "StageToPos.vi"("error in (no error)"=w305, "Move to pos"=w303, "Stage Select"=StageSelect."Y axis", "Device In"=w299) -> ("error out"=w301:errorcluster)  [unwired: 7 in]
                    n136 = Merge Errors(w302, w301) -> (w298:errorcluster)
                  }
                  frame #1 {
                    n137 = Wait (ms)(milliseconds to wait=u32 400) -> ()  [unwired: 1 out]
                  }
                }
                n138 = Wait (ms)(milliseconds to wait=u32 100) -> ()  [unwired: 1 out]
              }
              frame #2 {
                n139 = Subtract(x=w322, y=w321) -> (x-y=w324:i16)
                n140 = Subtract(x=w329, y=w328) -> (x-y=w327:i16)
                n141 = Divide(x=w324, y=i16 50) -> (x/y=w316:dbl)
                n142 = Divide(x=w327, y=i16 50) -> (x/y=w325:dbl)
                n143 = for {
                  N: w316 -> [w336]
                  tunnel: w325 -> [w330]
                  tunnel: w320 -> [w340]
                  tunnel: w319 -> [w339]
                  tunnel: w318 -> [w338]
                  tunnel: w317 -> [w337]
                  i -> [w333]
                  n144 = Round Toward -Infinity(1:w330) -> (0:→"Total_Frame_X":dbl)
                  n145 = Increment(x=w333) -> (x+1=→"Frame_Y":i32)
                  n146 = Divide(x=w333, y=2) -> (x/y=w345:dbl)
                  n147 = Round Toward -Infinity(1:w345) -> (0:w342:dbl)
                  n148 = Round Toward +Infinity(x=w345) -> (ceil(x): smallest int >= x=w343:dbl)
                  n149 = Equal?(x=w343, y=w342) -> (x = y?=w341:bool)
                  n150 = stacked-sequence {
                    tunnel: w341 -> [_ w358 w410]
                    tunnel: w330 -> [_ _ w409]
                    tunnel: w340 -> [w355 _ w408]
                    tunnel: w339 -> [_ w359 w407]
                    tunnel: w338 -> [_ w360 w406]
                    tunnel: w337 -> [_ w361 w405]
                    tunnel: w333 -> [_ w357 w404]
                    tunnel: w330 -> [_ w356 w403]
                    tunnel: [_ _ w402] -> w335
                    frame #0 {
                      w353 = 1 items=["Forward"=1, "Backward"=2] ("direction")
                      n151 = Unbundle By Name(w355) -> ("Device Y"=w354:refnum<k24>)  [unwired: 2 out]
                      n152 = Divide(x=0.0877 ("y"), y=1000.0) -> (x/y=w346:dbl)
                      n153 = Multiply(x=50.0, y=w346) -> (x*y=w349:dbl)
                      n154 = invoke class="KCubeDCServo" method="MoveRelative"(reference=w354, "direction"=w353, "stepSize"=w349, "waitTimeout"=0) -> ()  [unwired: 2 in, 6 out]
                      n155 = Wait (ms)(milliseconds to wait=u32 300) -> ()  [unwired: 1 out]
                    }
                    frame #1 {
                      n156 = case shown="False" w358 {
                        tunnel: w361 -> [w368 w387]
                        tunnel: w360 -> [w366 w386]
                        tunnel: w359 -> [w367 w385]
                        tunnel: w357 -> [w364 w383]
                        tunnel: w356 -> [w363 _]
                        frame False {
                          n157 = Round Toward -Infinity(1:w363) -> (0:w362:dbl)
                          n158 = Increment(x=w364) -> (x+1=w369:i32)
                          n159 = Number To Decimal String(number=w362) -> (decimal integer string=w365:string)  [unwired: 1 in]
                          n160 = Number To Decimal String(number=w369) -> (decimal integer string=w374:string)  [unwired: 1 in]
                          n161 = Concatenate Strings("x" ("string"), w365, "_y" ("string"), w374, ".png" ("string")) -> (w378:string)
                          n162 = Unbundle(w366) -> ("Height"=w372:i32, "Width"=w371:i32)
                          n163 = Build Path(base path=w368, name or relative path=w378) -> (appended path=w373:path)
                          n164 = call "GetActImgMem.vi"("Camera Handle In"=w367) -> ("Image Memory Out"=w381:u8[])  [unwired: 7 in, 3 out]
                          n165 = Reshape Array(w381, w372, w371) -> (w382:u8[][])
                          n166 = call <vilib>:"Flatten Pixmap.vi"("colors"=u32[] [0, 65793, 131586, 197379, 263172, 328965, 394758, 460551, 526344, 592137, 657930, 723723, 789516, 855309, 921102, 986895, 1052688, 1118481, 1184274, 1250067, 1315860, 1381653, 1447446, 1513239, 1579032, 1644825, 1710618, 1776411, 1842204, 1907997, 1973790, 2039583, 2105376, 2171169, 2236962, 2302755, 2368548, 2434341, 2500134, 2565927, 2631720, 2697513, 2763306, 2829099, 2894892, 2960685, 3026478, 3092271, 3158064, 3223857, 3289650, 3355443, 3421236, 3487029, 3552822, 3618615, 3684408, 3750201, 3815994, 3881787, 3947580, 4013373, 4079166, 4144959, 4210752, 4276545, 4342338, 4408131, 4473924, 4539717, 4605510, 4671303, 4737096, 4802889, 4868682, 4934475, 5000268, 5066061, 5131854, 5197647, 5263440, 5329233, 5395026, 5460819, 5526612, 5592405, 5658198, 5723991, 5789784, 5855577, 5921370, 5987163, 6052956, 6118749, 6184542, 6250335, 6316128, 6381921, 6447714, 6513507, 6579300, 6645093, 6710886, 6776679, 6842472, 6908265, 6974058, 7039851, 7105644, 7171437, 7237230, 7303023, 7368816, 7434609, 7500402, 7566195, 7631988, 7697781, 7763574, 7829367, 7895160, 7960953, 8026746, 8092539, 8158332, 8224125, 8289918, 8355711, 8421504, 8487297, 8553090, 8618883, 8684676, 8750469, 8816262, 8882055, 8947848, 9013641, 9079434, 9145227, 9211020, 9276813, 9342606, 9408399, 9474192, 9539985, 9605778, 9671571, 9737364, 9803157, 9868950, 9934743, 10000536, 10066329, 10132122, 10197915, 10263708, 10329501, 10395294, 10461087, 10526880, 10592673, 10658466, 10724259, 10790052, 10855845, 10921638, 10987431, 11053224, 11119017, 11184810, 11250603, 11316396, 11382189, 11447982, 11513775, 11579568, 11645361, 11711154, 11776947, 11842740, 11908533, 11974326, 12040119, 12105912, 12171705, 12237498, 12303291, 12369084, 12434877, 12500670, 12566463, 12632256, 12698049, 12763842, 12829635, 12895428, 12961221, 13027014, 13092807, 13158600, 13224393, 13290186, 13355979, 13421772, 13487565, 13553358, 13619151, 13684944, 13750737, 13816530, 13882323, 13948116, 14013909, 14079702, 14145495, 14211288, 14277081, 14342874, 14408667, 14474460, 14540253, 14606046, 14671839, 14737632, 14803425, 14869218, 14935011, 15000804, 15066597, 15132390, 15198183, 15263976, 15329769, 15395562, 15461355, 15527148, 15592941, 15658734, 15724527, 15790320, 15856113, 15921906, 15987699, 16053492, 16119285, 16185078, 16250871, 16316664, 16382457, 16448250, 16514043, 16579836, 16645629, 16711422, 0] ("output array 2"), "8-bit pixmap"=w382) -> ("image data"=w379:T13)  [unwired: 9 in]
                          n167 = Wait (ms)(milliseconds to wait=u32 300) -> ()  [unwired: 1 out]
                          n168 = call <vilib>:"Write PNG File.vi"("image data"=w379, "path to PNG file"=w373) -> ()  [unwired: 8 in, 2 out]
                        }
                        frame True {
                          n169 = Increment(x=w383) -> (x+1=w388:i32)
                          n170 = Number To Decimal String(number=w388) -> (decimal integer string=w393:string)  [unwired: 1 in]
                          n171 = Concatenate Strings("x" ("string"), "0" ("string"), "_y" ("string"), w393, ".png" ("string")) -> (w397:string)
                          n172 = Unbundle(w386) -> ("Height"=w391:i32, "Width"=w390:i32)
                          n173 = Build Path(base path=w387, name or relative path=w397) -> (appended path=w392:path)
                          n174 = call "GetActImgMem.vi"("Camera Handle In"=w385) -> ("Image Memory Out"=w400:u8[])  [unwired: 7 in, 3 out]
                          n175 = Reshape Array(w400, w391, w390) -> (w401:u8[][])
                          n176 = call <vilib>:"Flatten Pixmap.vi"("colors"=u32[] [0, 65793, 131586, 197379, 263172, 328965, 394758, 460551, 526344, 592137, 657930, 723723, 789516, 855309, 921102, 986895, 1052688, 1118481, 1184274, 1250067, 1315860, 1381653, 1447446, 1513239, 1579032, 1644825, 1710618, 1776411, 1842204, 1907997, 1973790, 2039583, 2105376, 2171169, 2236962, 2302755, 2368548, 2434341, 2500134, 2565927, 2631720, 2697513, 2763306, 2829099, 2894892, 2960685, 3026478, 3092271, 3158064, 3223857, 3289650, 3355443, 3421236, 3487029, 3552822, 3618615, 3684408, 3750201, 3815994, 3881787, 3947580, 4013373, 4079166, 4144959, 4210752, 4276545, 4342338, 4408131, 4473924, 4539717, 4605510, 4671303, 4737096, 4802889, 4868682, 4934475, 5000268, 5066061, 5131854, 5197647, 5263440, 5329233, 5395026, 5460819, 5526612, 5592405, 5658198, 5723991, 5789784, 5855577, 5921370, 5987163, 6052956, 6118749, 6184542, 6250335, 6316128, 6381921, 6447714, 6513507, 6579300, 6645093, 6710886, 6776679, 6842472, 6908265, 6974058, 7039851, 7105644, 7171437, 7237230, 7303023, 7368816, 7434609, 7500402, 7566195, 7631988, 7697781, 7763574, 7829367, 7895160, 7960953, 8026746, 8092539, 8158332, 8224125, 8289918, 8355711, 8421504, 8487297, 8553090, 8618883, 8684676, 8750469, 8816262, 8882055, 8947848, 9013641, 9079434, 9145227, 9211020, 9276813, 9342606, 9408399, 9474192, 9539985, 9605778, 9671571, 9737364, 9803157, 9868950, 9934743, 10000536, 10066329, 10132122, 10197915, 10263708, 10329501, 10395294, 10461087, 10526880, 10592673, 10658466, 10724259, 10790052, 10855845, 10921638, 10987431, 11053224, 11119017, 11184810, 11250603, 11316396, 11382189, 11447982, 11513775, 11579568, 11645361, 11711154, 11776947, 11842740, 11908533, 11974326, 12040119, 12105912, 12171705, 12237498, 12303291, 12369084, 12434877, 12500670, 12566463, 12632256, 12698049, 12763842, 12829635, 12895428, 12961221, 13027014, 13092807, 13158600, 13224393, 13290186, 13355979, 13421772, 13487565, 13553358, 13619151, 13684944, 13750737, 13816530, 13882323, 13948116, 14013909, 14079702, 14145495, 14211288, 14277081, 14342874, 14408667, 14474460, 14540253, 14606046, 14671839, 14737632, 14803425, 14869218, 14935011, 15000804, 15066597, 15132390, 15198183, 15263976, 15329769, 15395562, 15461355, 15527148, 15592941, 15658734, 15724527, 15790320, 15856113, 15921906, 15987699, 16053492, 16119285, 16185078, 16250871, 16316664, 16382457, 16448250, 16514043, 16579836, 16645629, 16711422, 0] ("output array 2"), "8-bit pixmap"=w401) -> ("image data"=w398:T13)  [unwired: 9 in]
                          n177 = Wait (ms)(milliseconds to wait=u32 300) -> ()  [unwired: 1 out]
                          n178 = call <vilib>:"Write PNG File.vi"("image data"=w398, "path to PNG file"=w392) -> ()  [unwired: 8 in, 2 out]
                        }
                      }
                    }
                    frame #2 {
                      n179 = case shown="False" w410 {
                        tunnel: w409 -> [w418 w467]
                        tunnel: w408 -> [w417 w466]
                        tunnel: w407 -> [w415 w465]
                        tunnel: w406 -> [w412 w464]
                        tunnel: w405 -> [w416 w463]
                        tunnel: w404 -> [w414 w462]
                        tunnel: w403 -> [w413 _]
                        tunnel: [w411 w461] -> w402
                        frame False {
                          n180 = for {
                            N: w418 -> [_]
                            tunnel: w417 -> [w425]
                            tunnel: w416 -> [w424]
                            tunnel: w415 -> [w423]
                            tunnel: w414 -> [w422]
                            tunnel: w413 -> [w421]
                            tunnel: w412 -> [w420]
                            tunnel: [w419] -> w411
                            i -> [w419]
                            n181 = stacked-sequence {
                              tunnel: w425 -> [_ w430 _]
                              tunnel: w424 -> [_ _ w449]
                              tunnel: w423 -> [_ _ w448]
                              tunnel: w422 -> [_ _ w443]
                              tunnel: w419 -> [_ _ w441]
                              tunnel: w421 -> [_ _ w440]
                              tunnel: w420 -> [_ _ w447]
                              frame #0 {
                                n182 = Wait (ms)(milliseconds to wait=u32 100) -> ()  [unwired: 1 out]
                              }
                              frame #1 {
                                w436 = 2 items=["Forward"=1, "Backward"=2] ("direction")
                                n183 = Unbundle By Name(w430) -> ("Device X"=w431:refnum<k24>)  [unwired: 2 out]
                                n184 = Divide(x=0.0877 ("y"), y=1000.0) -> (x/y=w428:dbl)
                                n185 = Multiply(x=50.0, y=w428) -> (x*y=w432:dbl)
                                n186 = invoke class="KCubeDCServo" method="MoveRelative"(reference=w431, "direction"=w436, "stepSize"=w432, "waitTimeout"=0) -> ()  [unwired: 2 in, 6 out]
                                n187 = Wait (ms)(milliseconds to wait=u32 450) -> ()  [unwired: 1 out]
                              }
                              frame #2 {
                                n188 = Round Toward -Infinity(1:w440) -> (0:w439:dbl)
                                n189 = Decrement(x=w439) -> (x-1=w438:dbl)
                                n190 = Subtract(x=w438, y=w441) -> (x-y=w437:dbl)
                                n191 = Increment(x=w443) -> (x+1=w442:i32)
                                n192 = Number To Decimal String(number=w437) -> (decimal integer string=w452:string)  [unwired: 1 in]
                                n193 = Number To Decimal String(number=w442) -> (decimal integer string=w451:string)  [unwired: 1 in]
                                n194 = Concatenate Strings("x" ("string"), w452, "_y" ("string"), w451, ".png" ("string")) -> (w456:string)
                                n195 = Unbundle(w447) -> ("Height"=w446:i32, "Width"=w445:i32)
                                n196 = Build Path(base path=w449, name or relative path=w456) -> (appended path=w450:path)
                                n197 = call "GetActImgMem.vi"("Camera Handle In"=w448) -> ("Image Memory Out"=w459:u8[])  [unwired: 7 in, 3 out]
                                n198 = Reshape Array(w459, w446, w445) -> (w460:u8[][])
                                n199 = call <vilib>:"Flatten Pixmap.vi"("colors"=u32[] [0, 65793, 131586, 197379, 263172, 328965, 394758, 460551, 526344, 592137, 657930, 723723, 789516, 855309, 921102, 986895, 1052688, 1118481, 1184274, 1250067, 1315860, 1381653, 1447446, 1513239, 1579032, 1644825, 1710618, 1776411, 1842204, 1907997, 1973790, 2039583, 2105376, 2171169, 2236962, 2302755, 2368548, 2434341, 2500134, 2565927, 2631720, 2697513, 2763306, 2829099, 2894892, 2960685, 3026478, 3092271, 3158064, 3223857, 3289650, 3355443, 3421236, 3487029, 3552822, 3618615, 3684408, 3750201, 3815994, 3881787, 3947580, 4013373, 4079166, 4144959, 4210752, 4276545, 4342338, 4408131, 4473924, 4539717, 4605510, 4671303, 4737096, 4802889, 4868682, 4934475, 5000268, 5066061, 5131854, 5197647, 5263440, 5329233, 5395026, 5460819, 5526612, 5592405, 5658198, 5723991, 5789784, 5855577, 5921370, 5987163, 6052956, 6118749, 6184542, 6250335, 6316128, 6381921, 6447714, 6513507, 6579300, 6645093, 6710886, 6776679, 6842472, 6908265, 6974058, 7039851, 7105644, 7171437, 7237230, 7303023, 7368816, 7434609, 7500402, 7566195, 7631988, 7697781, 7763574, 7829367, 7895160, 7960953, 8026746, 8092539, 8158332, 8224125, 8289918, 8355711, 8421504, 8487297, 8553090, 8618883, 8684676, 8750469, 8816262, 8882055, 8947848, 9013641, 9079434, 9145227, 9211020, 9276813, 9342606, 9408399, 9474192, 9539985, 9605778, 9671571, 9737364, 9803157, 9868950, 9934743, 10000536, 10066329, 10132122, 10197915, 10263708, 10329501, 10395294, 10461087, 10526880, 10592673, 10658466, 10724259, 10790052, 10855845, 10921638, 10987431, 11053224, 11119017, 11184810, 11250603, 11316396, 11382189, 11447982, 11513775, 11579568, 11645361, 11711154, 11776947, 11842740, 11908533, 11974326, 12040119, 12105912, 12171705, 12237498, 12303291, 12369084, 12434877, 12500670, 12566463, 12632256, 12698049, 12763842, 12829635, 12895428, 12961221, 13027014, 13092807, 13158600, 13224393, 13290186, 13355979, 13421772, 13487565, 13553358, 13619151, 13684944, 13750737, 13816530, 13882323, 13948116, 14013909, 14079702, 14145495, 14211288, 14277081, 14342874, 14408667, 14474460, 14540253, 14606046, 14671839, 14737632, 14803425, 14869218, 14935011, 15000804, 15066597, 15132390, 15198183, 15263976, 15329769, 15395562, 15461355, 15527148, 15592941, 15658734, 15724527, 15790320, 15856113, 15921906, 15987699, 16053492, 16119285, 16185078, 16250871, 16316664, 16382457, 16448250, 16514043, 16579836, 16645629, 16711422, 0] ("output array 2"), "8-bit pixmap"=w460) -> ("image data"=w457:T13)  [unwired: 9 in]
                                n200 = Wait (ms)(milliseconds to wait=u32 300) -> ()  [unwired: 1 out]
                                n201 = call <vilib>:"Write PNG File.vi"("image data"=w457, "path to PNG file"=w450) -> ()  [unwired: 8 in, 2 out]
                              }
                            }
                          }
                        }
                        frame True {
                          n202 = for {
                            N: w467 -> [_]
                            tunnel: w466 -> [w473]
                            tunnel: w465 -> [w472]
                            tunnel: w464 -> [w471]
                            tunnel: w463 -> [w470]
                            tunnel: w462 -> [w469]
                            tunnel: [w468] -> w461
                            i -> [w468]
                            n203 = stacked-sequence {
                              tunnel: w473 -> [_ w479 _]
                              tunnel: w472 -> [_ _ w499]
                              tunnel: w471 -> [_ _ w498]
                              tunnel: w470 -> [_ _ w496]
                              tunnel: w468 -> [_ _ w486]
                              tunnel: w469 -> [_ _ w488]
                              frame #0 {
                                n204 = Wait (ms)(milliseconds to wait=u32 100) -> ()  [unwired: 1 out]
                              }
                              frame #1 {
                                w484 = 1 items=["Forward"=1, "Backward"=2] ("direction")
                                n205 = Unbundle By Name(w479) -> ("Device X"=w478:refnum<k24>)  [unwired: 2 out]
                                n206 = Divide(x=0.0877 ("y"), y=1000.0) -> (x/y=w475:dbl)
                                n207 = Multiply(x=50.0, y=w475) -> (x*y=w480:dbl)
                                n208 = invoke class="KCubeDCServo" method="MoveRelative"(reference=w478, "direction"=w484, "stepSize"=w480, "waitTimeout"=0) -> ()  [unwired: 2 in, 6 out]
                                n209 = Wait (ms)(milliseconds to wait=u32 400) -> ()  [unwired: 1 out]
                              }
                              frame #2 {
                                n210 = Increment(x=w486) -> (x+1=w485:i32)
                                n211 = Increment(x=w488) -> (x+1=w487:i32)
                                n212 = Number To Decimal String(number=w487) -> (decimal integer string=w491:string)  [unwired: 1 in]
                                n213 = Number To Decimal String(number=w485) -> (decimal integer string=w492:string)  [unwired: 1 in]
                                n214 = Concatenate Strings("x" ("string"), w492, "_y" ("string"), w491, ".png" ("string")) -> (w497:string)
                                n215 = Build Path(base path=w496, name or relative path=w497) -> (appended path=w490:path)
                                n216 = call "GetActImgMem.vi"("Camera Handle In"=w499) -> ("Image Memory Out"=w502:u8[])  [unwired: 7 in, 3 out]
                                n217 = Unbundle(w498) -> ("Height"=w503:i32, "Width"=w504:i32)
                                n218 = Reshape Array(w502, w503, w504) -> (w505:u8[][])
                                n219 = call <vilib>:"Flatten Pixmap.vi"("colors"=u32[] [0, 65793, 131586, 197379, 263172, 328965, 394758, 460551, 526344, 592137, 657930, 723723, 789516, 855309, 921102, 986895, 1052688, 1118481, 1184274, 1250067, 1315860, 1381653, 1447446, 1513239, 1579032, 1644825, 1710618, 1776411, 1842204, 1907997, 1973790, 2039583, 2105376, 2171169, 2236962, 2302755, 2368548, 2434341, 2500134, 2565927, 2631720, 2697513, 2763306, 2829099, 2894892, 2960685, 3026478, 3092271, 3158064, 3223857, 3289650, 3355443, 3421236, 3487029, 3552822, 3618615, 3684408, 3750201, 3815994, 3881787, 3947580, 4013373, 4079166, 4144959, 4210752, 4276545, 4342338, 4408131, 4473924, 4539717, 4605510, 4671303, 4737096, 4802889, 4868682, 4934475, 5000268, 5066061, 5131854, 5197647, 5263440, 5329233, 5395026, 5460819, 5526612, 5592405, 5658198, 5723991, 5789784, 5855577, 5921370, 5987163, 6052956, 6118749, 6184542, 6250335, 6316128, 6381921, 6447714, 6513507, 6579300, 6645093, 6710886, 6776679, 6842472, 6908265, 6974058, 7039851, 7105644, 7171437, 7237230, 7303023, 7368816, 7434609, 7500402, 7566195, 7631988, 7697781, 7763574, 7829367, 7895160, 7960953, 8026746, 8092539, 8158332, 8224125, 8289918, 8355711, 8421504, 8487297, 8553090, 8618883, 8684676, 8750469, 8816262, 8882055, 8947848, 9013641, 9079434, 9145227, 9211020, 9276813, 9342606, 9408399, 9474192, 9539985, 9605778, 9671571, 9737364, 9803157, 9868950, 9934743, 10000536, 10066329, 10132122, 10197915, 10263708, 10329501, 10395294, 10461087, 10526880, 10592673, 10658466, 10724259, 10790052, 10855845, 10921638, 10987431, 11053224, 11119017, 11184810, 11250603, 11316396, 11382189, 11447982, 11513775, 11579568, 11645361, 11711154, 11776947, 11842740, 11908533, 11974326, 12040119, 12105912, 12171705, 12237498, 12303291, 12369084, 12434877, 12500670, 12566463, 12632256, 12698049, 12763842, 12829635, 12895428, 12961221, 13027014, 13092807, 13158600, 13224393, 13290186, 13355979, 13421772, 13487565, 13553358, 13619151, 13684944, 13750737, 13816530, 13882323, 13948116, 14013909, 14079702, 14145495, 14211288, 14277081, 14342874, 14408667, 14474460, 14540253, 14606046, 14671839, 14737632, 14803425, 14869218, 14935011, 15000804, 15066597, 15132390, 15198183, 15263976, 15329769, 15395562, 15461355, 15527148, 15592941, 15658734, 15724527, 15790320, 15856113, 15921906, 15987699, 16053492, 16119285, 16185078, 16250871, 16316664, 16382457, 16448250, 16514043, 16579836, 16645629, 16711422, 0] ("output array 2"), "8-bit pixmap"=w505) -> ("image data"=w500:T13)  [unwired: 9 in]
                                n220 = call <vilib>:"Write PNG File.vi"("image data"=w500, "path to PNG file"=w490) -> ()  [unwired: 8 in, 2 out]
                                n221 = Wait (ms)(milliseconds to wait=u32 300) -> ()  [unwired: 1 out]
                              }
                            }
                          }
                        }
                      }
                    }
                  }
                  n222 = Increment(x=w335) -> (x+1=→"Frame_X":i32)
                  "Total_Frame_Y" <- w336
                }
              }
              frame #3 {
                n223 = One Button Dialog(message="Scanning is finished!!!", button name ("OK")="OK") -> ()  [unwired: 1 out]
              }
            }
          }
          event "X axis_R": Value Change {
            n224 = event-data() -> ()  [unwired: 1 in, 6 out]
            n225 = Unbundle(w517) -> ("Device Y"=w515:refnum<k24>)  [unwired: 1 out]
            n226 = case shown="\"0.05mm\"" w509 {
              tunnel: [0.01 0.1 0.5 1.0 1.5 0.05] -> w508
              frame "0.01mm", Default {
              }
              frame "0.1mm" {
              }
              frame "0.5mm" {
              }
              frame "1mm" {
              }
              frame "1.5mm" {
              }
              frame "0.05mm" {
              }
            }
            n227 = Subtract(x=12.0, y=w508) -> (x-y=w513:dbl)
            n228 = Greater?(x=w513, y=w512) -> (0:w511:bool)
            n229 = case shown="True" w511 {
              tunnel: w515 -> [_ w529]
              tunnel: w508 -> [_ w528]
              frame False {
              }
              frame True {
                w531 = 1 items=["Forward"=1, "Backward"=2] ("direction")
                n230 = invoke class="KCubeDCServo" method="MoveRelative"(reference=w529, "direction"=w531, "stepSize"=w528, "waitTimeout"=0) -> ()  [unwired: 2 in, 6 out]
              }
            }
            n231 = Wait (ms)(milliseconds to wait=u32 50) -> ()  [unwired: 1 out]
          }
          event "X axis_L": Value Change {
            n232 = event-data() -> ()  [unwired: 1 in, 6 out]
            n233 = Unbundle(w538) -> ("Device Y"=w537:refnum<k24>)  [unwired: 1 out]
            n234 = case shown="\"0.05mm\"" w533 {
              tunnel: [0.01 0.1 0.5 1.0 1.5 0.05] -> w532
              frame "0.01mm", Default {
              }
              frame "0.1mm" {
              }
              frame "0.5mm" {
              }
              frame "1mm" {
              }
              frame "1.5mm" {
              }
              frame "0.05mm" {
              }
            }
            n235 = Less?(x=w532, y=w536) -> (x < y?=w535:bool)
            n236 = case shown="True" w535 {
              tunnel: w537 -> [_ w551]
              tunnel: w532 -> [_ w550]
              frame False {
              }
              frame True {
                w553 = 2 items=["Forward"=1, "Backward"=2] ("direction")
                n237 = invoke class="KCubeDCServo" method="MoveRelative"(reference=w551, "direction"=w553, "stepSize"=w550, "waitTimeout"=0) -> ()  [unwired: 2 in, 6 out]
              }
            }
            n238 = Wait (ms)(milliseconds to wait=u32 50) -> ()  [unwired: 1 out]
          }
          event "Y axis_B": Value Change {
            n239 = event-data() -> ()  [unwired: 1 in, 6 out]
            n240 = Unbundle(w560) -> ("Device Y"=w554:refnum<k24>)  [unwired: 1 out]
            n241 = case shown="\"0.05mm\"" w556 {
              tunnel: [0.01 0.1 0.5 1.0 1.5 0.05] -> w555
              frame "0.01mm", Default {
              }
              frame "0.1mm" {
              }
              frame "0.5mm" {
              }
              frame "1mm" {
              }
              frame "1.5mm" {
              }
              frame "0.05mm" {
              }
            }
            n242 = Subtract(x=12.0, y=w555) -> (x-y=w561:dbl)
            n243 = Greater?(x=w561, y=w558) -> (0:w559:bool)
            n244 = case shown="True" w559 {
              tunnel: w554 -> [_ w575]
              tunnel: w555 -> [_ w574]
              frame False {
              }
              frame True {
                w577 = 1 items=["Forward"=1, "Backward"=2] ("direction")
                n245 = invoke class="KCubeDCServo" method="MoveRelative"(reference=w575, "direction"=w577, "stepSize"=w574, "waitTimeout"=0) -> ()  [unwired: 2 in, 6 out]
              }
            }
            n246 = Wait (ms)(milliseconds to wait=u32 50) -> ()  [unwired: 1 out]
          }
          event "Y axis_F": Value Change {
            n247 = event-data() -> ()  [unwired: 1 in, 6 out]
            n248 = Unbundle(w583) -> (w582)  [unwired: 2 out]
            n249 = case shown="\"0.05mm\"" w579 {
              tunnel: [0.01 0.1 0.5 1.0 1.5 0.05] -> w578
              frame "0.01mm", Default {
              }
              frame "0.1mm" {
              }
              frame "0.5mm" {
              }
              frame "1mm" {
              }
              frame "1.5mm" {
              }
              frame "0.05mm" {
              }
            }
            n250 = Less?(x=w578, y=w581) -> (x < y?=w584:bool)
            n251 = case shown="True" w584 {
              tunnel: w582 -> [_ w597]
              tunnel: w578 -> [_ w596]
              frame False {
              }
              frame True {
                w599 = 2 items=["Forward"=1, "Backward"=2] ("direction")
                n252 = invoke class="KCubeDCServo" method="MoveRelative"(reference=w597, "direction"=w599, "stepSize"=w596, "waitTimeout"=0) -> ()  [unwired: 2 in, 6 out]
              }
            }
            n253 = Wait (ms)(milliseconds to wait=u32 50) -> ()  [unwired: 1 out]
          }
          event "Z axis_u": Value Change {
            n254 = event-data() -> ()  [unwired: 1 in, 6 out]
            n255 = Unbundle(w605) -> ("Device X"=w604:refnum<k24>)  [unwired: 1 out]
            n256 = case shown="\"20step\"" w606 {
              tunnel: [1 5 10 30 300 3000] -> w607
              frame "1step", Default {
              }
              frame "2step" {
              }
              frame "5step" {
              }
              frame "10step" {
              }
              frame "15step" {
              }
              frame "20step" {
              }
            }
            n257 = invoke class="KCubeDCServo" method="SetJogStepSize_DeviceUnit"(reference=w604, "stepSize"=w607) -> (reference out=w601:refnum<k24>)  [unwired: 2 in, 3 out]
            n258 = Less?(x=w602, y=11.5) -> (x < y?=w603:bool)
            n259 = case shown="True" w603 {
              tunnel: w601 -> [_ w614]
              frame False {
              }
              frame True {
                w616 = 1 items=["Forward"=1, "Backward"=2] ("direction")
                n260 = invoke class="KCubeDCServo" method="MoveJog"(reference=w614, "direction"=w616, "waitTimeout"=0) -> ()  [unwired: 2 in, 5 out]
              }
            }
            n261 = Wait (ms)(milliseconds to wait=u32 50) -> ()  [unwired: 1 out]
          }
          event "Z axis_d": Value Change {
            n262 = event-data() -> ()  [unwired: 1 in, 6 out]
            n263 = Unbundle(w629) -> ("Device X"=w630:refnum<k24>)  [unwired: 1 out]
            n264 = case shown="\"20step\"" w628 {
              tunnel: [1 5 10 30 300 3000] -> w631
              frame "1step", Default {
              }
              frame "2step" {
              }
              frame "5step" {
              }
              frame "10step" {
              }
              frame "15step" {
              }
              frame "20step" {
              }
            }
            n265 = invoke class="KCubeDCServo" method="SetJogStepSize_DeviceUnit"(reference=w630, "stepSize"=w631) -> (reference out=w627:refnum<k24>)  [unwired: 2 in, 3 out]
            n266 = Less?(x=0.01 ("y"), y=w625) -> (x < y?=w626:bool)
            n267 = case shown="True" w626 {
              tunnel: w627 -> [_ w637]
              frame False {
              }
              frame True {
                w639 = 2 items=["Forward"=1, "Backward"=2] ("direction")
                n268 = invoke class="KCubeDCServo" method="MoveJog"(reference=w637, "direction"=w639, "waitTimeout"=0) -> ()  [unwired: 2 in, 5 out]
              }
            }
            n269 = Wait (ms)(milliseconds to wait=u32 50) -> ()  [unwired: 1 out]
          }
          event "MoveTo": Value Change {
            n270 = event-data() -> ()  [unwired: 1 in, 6 out]
            n271 = Unbundle(w647) -> ("Device X"=w646:refnum<k24>)  [unwired: 1 out]
            n272 = invoke class="KCubeDCServo" method="MoveTo"(reference=w646, "position"="Destination", "waitTimeout"=0) -> ()  [unwired: 2 in, 5 out]
            n273 = Wait (ms)(milliseconds to wait=u32 1000) -> ()  [unwired: 1 out]
          }
          event "Snap": Value Change {
            n274 = event-data() -> ()  [unwired: 1 in, 6 out]
            n275 = call "GetActImgMem.vi"("Camera Handle In"=w665) -> ("Image Memory Out"=w660:u8[])  [unwired: 7 in, 3 out]
            n276 = Unbundle(w658) -> ("Height"=w661:i32, "Width"=w662:i32)
            n277 = Reshape Array(w660, w661, w662) -> (w663:u8[][])
            n278 = call <vilib>:"Flatten Pixmap.vi"("colors"=u32[] [0, 65793, 131586, 197379, 263172, 328965, 394758, 460551, 526344, 592137, 657930, 723723, 789516, 855309, 921102, 986895, 1052688, 1118481, 1184274, 1250067, 1315860, 1381653, 1447446, 1513239, 1579032, 1644825, 1710618, 1776411, 1842204, 1907997, 1973790, 2039583, 2105376, 2171169, 2236962, 2302755, 2368548, 2434341, 2500134, 2565927, 2631720, 2697513, 2763306, 2829099, 2894892, 2960685, 3026478, 3092271, 3158064, 3223857, 3289650, 3355443, 3421236, 3487029, 3552822, 3618615, 3684408, 3750201, 3815994, 3881787, 3947580, 4013373, 4079166, 4144959, 4210752, 4276545, 4342338, 4408131, 4473924, 4539717, 4605510, 4671303, 4737096, 4802889, 4868682, 4934475, 5000268, 5066061, 5131854, 5197647, 5263440, 5329233, 5395026, 5460819, 5526612, 5592405, 5658198, 5723991, 5789784, 5855577, 5921370, 5987163, 6052956, 6118749, 6184542, 6250335, 6316128, 6381921, 6447714, 6513507, 6579300, 6645093, 6710886, 6776679, 6842472, 6908265, 6974058, 7039851, 7105644, 7171437, 7237230, 7303023, 7368816, 7434609, 7500402, 7566195, 7631988, 7697781, 7763574, 7829367, 7895160, 7960953, 8026746, 8092539, 8158332, 8224125, 8289918, 8355711, 8421504, 8487297, 8553090, 8618883, 8684676, 8750469, 8816262, 8882055, 8947848, 9013641, 9079434, 9145227, 9211020, 9276813, 9342606, 9408399, 9474192, 9539985, 9605778, 9671571, 9737364, 9803157, 9868950, 9934743, 10000536, 10066329, 10132122, 10197915, 10263708, 10329501, 10395294, 10461087, 10526880, 10592673, 10658466, 10724259, 10790052, 10855845, 10921638, 10987431, 11053224, 11119017, 11184810, 11250603, 11316396, 11382189, 11447982, 11513775, 11579568, 11645361, 11711154, 11776947, 11842740, 11908533, 11974326, 12040119, 12105912, 12171705, 12237498, 12303291, 12369084, 12434877, 12500670, 12566463, 12632256, 12698049, 12763842, 12829635, 12895428, 12961221, 13027014, 13092807, 13158600, 13224393, 13290186, 13355979, 13421772, 13487565, 13553358, 13619151, 13684944, 13750737, 13816530, 13882323, 13948116, 14013909, 14079702, 14145495, 14211288, 14277081, 14342874, 14408667, 14474460, 14540253, 14606046, 14671839, 14737632, 14803425, 14869218, 14935011, 15000804, 15066597, 15132390, 15198183, 15263976, 15329769, 15395562, 15461355, 15527148, 15592941, 15658734, 15724527, 15790320, 15856113, 15921906, 15987699, 16053492, 16119285, 16185078, 16250871, 16316664, 16382457, 16448250, 16514043, 16579836, 16645629, 16711422, 0] ("output array 2"), "8-bit pixmap"=w663) -> ("image data"=w657:T13)  [unwired: 9 in]
            n279 = call <vilib>:"Write PNG File.vi"("image data"=w657) -> ()  [unwired: 9 in, 2 out]
          }
          event "Live video": Mouse Down {
            # "When the mouse is inside the video area, after the mouse is down and hold, the coordinate of the ROI upper left corner is stored."
            n280 = event-data() -> ("Coords"=w672:T5)  [unwired: 1 in, 7 out]
          }
          event "Live video": Mouse Up {
            # "When the mouse is inside the video area, after the mouse is up, the edge of the ROI is calculated."
            n281 = event-data() -> ("Coords"=w680:T5)  [unwired: 1 in, 7 out]
            n282 = property on="Live video" class="Pict"() -> ("Position"=w678:T14)  [unwired: 2 in, 2 out]
            n283 = Unbundle By Name "Start"(w679) -> ("Horizontal"=w700:i32, "Vertical"=w697:i32)
            n284 = Unbundle By Name(w680) -> ("Horizontal"=w694:i32, "Vertical"=w691:i32)
            n285 = Unbundle By Name(w678) -> ("Left"=w702:i32, "Top"=w701:i32)
            n286 = Subtract(x=w700, y=3) -> (x-y=w698:i32)
            n287 = Subtract(x=w697, y=3) -> (x-y=w696:i32)
            n288 = Subtract(x=w694, y=3) -> (x-y=w692:i32)
            n289 = Subtract(x=w691, y=3) -> (x-y=w689:i32)
            n290 = Subtract(x=w698, y=w702) -> (x-y=w688:i32)
            n291 = Subtract(x=w696, y=w701) -> (x-y=w687:i32)
            n292 = Subtract(x=w692, y=w702) -> (x-y=w675:i32)
            n293 = Subtract(x=w689, y=w701) -> (x-y=w674:i32)
            n294 = Divide(x=w688, y=w681) -> (x/y=w686:dbl)
            n295 = Divide(x=w687, y=w681) -> (x/y=w685:dbl)
            n296 = Divide(x=w675, y=w681) -> (x/y=w684:dbl)
            n297 = Divide(x=w674, y=w681) -> (x/y=w683:dbl)
            n298 = Bundle By Name(cluster=T4 {"left"=0, "top"=0, "right"=0, "bottom"=0} ("rect"), "left"=w686, "top"=w685, "right"=w684, "bottom"=w683) -> (w682:T4)
          }
          event "Quit": Value Change {
            # "Add recover initial position\nZ: max\nX: middle\nY: middle\nand also need to attch a limit"
            # "When user clicks the STOP button, program will jump to \"Shut down\" state"
            n299 = event-data() -> ()  [unwired: 1 in, 6 out]
          }
          event "Aim": Value Change {
            # "First, you need to draw an ROI, and then when you click the Aim button, the center of the\nview will move to the center of the selected ROI."
            n300 = event-data() -> ()  [unwired: 1 in, 6 out]
            n301 = Unbundle By Name(w746) -> ("left"=w744:i16, "right"=w745:i16, "top"=w739:i16, "bottom"=w738:i16)
            n302 = Unbundle By Name(w712) -> ("Laser X"=w711:dbl, "Laser Y"=w710:dbl)
            n303 = Add(x=w744, y=w745) -> (x+y=w743:i16)
            n304 = Add(x=w739, y=w738) -> (x+y=w740:i16)
            n305 = Divide(x=w743, y=i16 2) -> (x/y=w737:dbl)
            n306 = Divide(x=w740, y=i16 2) -> (x/y=w736:dbl)
            n307 = Subtract(x=w737, y=w711) -> (x-y=w726:dbl)
            n308 = Subtract(x=w736, y=w710) -> (x-y=w731:dbl)
            n309 = Divide(x="Pixel Size Y (um)", y=1000.0) -> (x/y=w727:dbl)
            n310 = Divide(x="Pixel Size X (um)", y=1000.0) -> (x/y=w725:dbl)
            n311 = Multiply(x=w725, y=w726) -> (x*y=w732:dbl)
            n312 = Multiply(x=w731, y=w727) -> (x*y=w730:dbl)
            n313 = call "StageReadPos.vi"("error in (no error)"=w747, "Stage Select"=StageSelect."X axis", "Device In"=w735) -> ("error out"=w724:errorcluster, "CurrentPosition"=w721:dbl)  [unwired: 7 in]
            n314 = call "StageReadPos.vi"("error in (no error)"=w747, "Stage Select"=StageSelect."Y axis", "Device In"=w735) -> ("error out"=w717:errorcluster, "CurrentPosition"=w716:dbl)  [unwired: 7 in]
            n315 = Add(x=w730, y=w716) -> (x+y=w715:dbl)
            n316 = Add(x=w732, y=w721) -> (x+y=w720:dbl)
            n317 = call "StageToPos.vi"("error in (no error)"=w724, "Move to pos"=w720, "Stage Select"=StageSelect."X axis", "Device In"=w735) -> ("error out"=w714:errorcluster)  [unwired: 7 in]
            n318 = call "StageToPos.vi"("error in (no error)"=w717, "Move to pos"=w715, "Stage Select"=StageSelect."Y axis", "Device In"=w735) -> ("error out"=w713:errorcluster)  [unwired: 7 in]
            n319 = Merge Errors(w714, w713) -> (w748:errorcluster)
          }
          event "LaserSpot": Value Change {
            # "First, you need to draw an ROI, and then when you click the Here's Laser button, the center of the\nROI will be stored for Aim use."
            n320 = event-data() -> ()  [unwired: 1 in, 6 out]
            n321 = Unbundle By Name(w756) -> ("left"=w763:i16, "right"=w764:i16, "top"=w758:i16, "bottom"=w757:i16)
            n322 = Add(x=w763, y=w764) -> (x+y=w762:i16)
            n323 = Add(x=w758, y=w757) -> (x+y=w759:i16)
            n324 = Divide(x=w762, y=i16 2) -> (x/y=w752:dbl)
            n325 = Divide(x=w759, y=i16 2) -> (x/y=w751:dbl)
            n326 = Bundle By Name(cluster=T3 {"Laser X"=0.0, "Laser Y"=0.0} ("LaserSpot"), "Laser X"=w752, "Laser Y"=w751) -> (w754:T3)
            n327 = local write "Spot Y"(w751) -> ()
            n328 = local write "Spot X"(w752) -> ()
            "Boolean" <- TRUE ("Boolean")
          }
          event "Left": Value Change {
            n329 = event-data() -> ()  [unwired: 1 in, 6 out]
            n330 = Unbundle By Name(w771) -> ("Laser X"=w769:dbl, "Laser Y"=w770:dbl)
            n331 = Decrement(x=w769) -> (x-1=w768:dbl)
            n332 = Bundle By Name(cluster=T3 {"Laser X"=0.0, "Laser Y"=0.0} ("LaserSpot"), "Laser X"=w768, "Laser Y"=w770) -> (w772:T3)
            n333 = local write "Spot X"(w768) -> ()
          }
          event "Right": Value Change {
            n334 = event-data() -> ()  [unwired: 1 in, 6 out]
            n335 = Unbundle By Name(w781) -> ("Laser X"=w779:dbl, "Laser Y"=w782:dbl)
            n336 = Increment(x=w779) -> (x+1=w778:dbl)
            n337 = Bundle By Name(cluster=T3 {"Laser X"=0.0, "Laser Y"=0.0} ("LaserSpot"), "Laser X"=w778, "Laser Y"=w782) -> (w780:T3)
            n338 = local write "Spot X"(w778) -> ()
          }
          event "Top": Value Change {
            n339 = event-data() -> ()  [unwired: 1 in, 6 out]
            n340 = Unbundle By Name(w792) -> ("Laser X"=w790:dbl, "Laser Y"=w789:dbl)
            n341 = Decrement(x=w789) -> (x-1=w788:dbl)
            n342 = Bundle By Name(cluster=T3 {"Laser X"=0.0, "Laser Y"=0.0} ("LaserSpot"), "Laser X"=w790, "Laser Y"=w788) -> (w791:T3)
            n343 = local write "Spot Y"(w788) -> ()
          }
          event "Down": Value Change {
            n344 = event-data() -> ()  [unwired: 1 in, 6 out]
            n345 = Unbundle By Name(w802) -> ("Laser X"=w800:dbl, "Laser Y"=w799:dbl)
            n346 = Increment(x=w799) -> (x+1=w798:dbl)
            n347 = Bundle By Name(cluster=T3 {"Laser X"=0.0, "Laser Y"=0.0} ("LaserSpot"), "Laser X"=w800, "Laser Y"=w798) -> (w801:T3)
            n348 = local write "Spot Y"(w798) -> ()
          }
        }
      }
    }
  }
  n349 = call <vilib>:"Simple Error Handler.vi"("error in (no error)"=w9) -> ()  [unwired: 4 in, 5 out]
